vi "v3.vi"() -> ()   [LabVIEW 2015]
uses:
  <vilib>/Utility/miscctls.llb/LVDateTimeRec.ctl
  <vilib>/Analysis/3filter.llb/Filter Passband Type.ctl
  <vilib>/Analysis/8numeric.llb/1D Numeric Integration.vi
  <vilib>/Utility/inputDevices.llb/mouseAcquire.vi
  <vilib>/Utility/inputDevices.llb/closeMouse.vi
  <vilib>/Utility/cursorutil.llb/Set Cursor (Icon Pict).vi
  <vilib>/Analysis/3filter.llb/Butterworth Filter (DBL).vi
  <vilib>/Utility/file.llb/Write Delimited Spreadsheet (DBL).vi
  <vilib>/Analysis/NI_AALBase.lvlib
  <vilib>/Analysis/NI_AALPro.lvlib
panel:
  out "ER":string
  out "TM":string
  out "Vertical (cm/px)":dbl
  out "Horizontal (cm/px)":dbl
  out "Alvo_vertical_px":dbl
  out "Alvo_horizontal_px":dbl
  out "Horizontal_atual_px":i32
  out "Vertical_atual_px":i32
  out "cont6":dbl
  out "cont5":dbl
  out "cont4":dbl
  out "cont2":dbl
  out "cont3":dbl
  out "cont1":dbl
  out "codigo":dbl
  out "Area_acel_1_sub":dbl format="%0.4f"
  out "Area_acel_2_sub":dbl format="%0.4f"
  out "Posicao_final_horizontal":dbl
  out "Posicao_final_Vertical":dbl
  out "Posicao_Hori_2_sub":dbl
  out "Posicao_vert_2_sub":dbl
  out "Deslocamento_Horizontal_fill":dbl[](array[numeric])
  out "Deslocamento_Vertical_fill":dbl[](array[numeric])
  out "Deslocamento_tototal_1_sub":dbl[](array[numeric])
  out "Deslocamento_tototal_2_sub":dbl[](array[numeric])
  out "2_sub_mov(s)":dbl
  out "Fim_da_reposta(s)":dbl format="%#.17g"
  out "Inicio_da_reposta(s)":dbl format="%#.17g"
  out "Apresentacao_do_estimulo(s)":dbl format="%#.17g"
  out "Fim_do_warning(s)":dbl format="%#.17g"
  out "Inicio_do_warning(s)":dbl format="%#.17g"
  out "INICIO(s)":dbl format="%#.17g"
  out "Fim_resp_Cluter":T1
  out "Inicio_da_resposta_Cluter":T1
  out "Apresentacao_do_estimulo_Cluter":T1
  out "Fim_do_warning_Cluter":T1
  out "Inicio_do_warning_Cluter":T1
  out "INICIO_Cluter":T1
  out "x/y":dbl
  out "Fim_do_warning":dbl format="%#.10g"
  out "Inicio_do_warning":dbl format="%#.10g"
  out "Posicao_graus_2_sub":dbl
  out "Posicao_cm_2_sub":dbl
  out "ER_no_2_sub":dbl
  out "Posicao_cm_final":dbl
  out "2_sub_mov":dbl format="%#.10g"
  out "Posicao_graus_final":dbl
  out "Graus":dbl[](array[numeric])
  out "n_correcoes":i32
  out "ref_zero_cross":i32[](array[numeric])
  out "Tempo_relativo_pico":dbl
  out "Tempo_para_o_pico":i32
  out "Pico_velocidade":dbl
  out "Fim_resp":dbl format="%#.10g"
  out "Inicio_da_resposta":dbl format="%#.10g"
  out "Vertical_posicao_px":i32[](array[numeric])
  out "Horizontal_posicao_px":i32[](array[numeric])
  out "Jeark":dbl[](array[numeric])
  out "Deslocamento_Horizontal_bruto":dbl[](array[numeric])
  out "Deslocamento_Vertical_bruto":dbl[](array[numeric])
  out "ref_p_inicial_vertical":dbl
  out "posicao_total":dbl[](array[numeric])
  out "INICIO":dbl format="%#.10g"
  out "Apresentacao_do_estimulo":dbl format="%#.10g"
  out "ref_p_inicial_total":dbl
  out "posicao_horizontal":dbl[](array[numeric])
  out "posicao_vertical":dbl[](array[numeric])
  out "Array_x":dbl[](array[numeric])
  out "ref_t_max":dbl
  out "ref_TR":i32
  out "erro radial (cm)":dbl
  out "meta_precisao":dbl
  out "ref_V_alvo":dbl
  out "ref_H_alvo":dbl
  out "ponto_final":dbl
  out "ref_pont":dbl
  out "Deslocamento_Total__bruto":dbl[](array[numeric])
  out "tentativa":i32
  out "referencia de endereco":path
  out "aceleracao":dbl[](array[numeric])
  out "Velocidade":dbl[](array[numeric])
  out "eixo x":dbl[](array[numeric])
  out "Deslocamento_total_filtrado":dbl[](array[numeric])
  out "cursor":picture
  in  "Tab Control":enum32{"Execucao", "Configuração", "Gráficos"}(tab)
  out "tela":picture
  out "ref_p_inicial_horizontal":dbl
  in  "Cor do ponteiro":u32(colorbox)=14421504
  in  "Cor":u32(colorbox)=197379
  in  "Cor":u32(colorbox)
  in  "Tempo do warning estimulo":u32=1000
  in  "Maior":dbl=3000.0
  in  "menor":dbl=1000.0 format="%#_13g"
  in  "Intervalo entre o fim e o inicio da próxima tentativa":u32=500
  in  "Horizontal (px)":dbl=1366.0
  in  "Horizontal (cm)":dbl=47.2
  in  "Raio":dbl=1.0
  in  "Horizontal":dbl=11.0
  in  "Vertical":dbl=20.0
  in  "Raio":dbl
  in  "Horizontal":dbl
  in  "Vertical":dbl
  in  "Tamanho do ponteiro":dbl=0.2
  in  "Cor":u32(colorbox)
  in  "Raio":dbl
  in  "Horizontal":dbl
  in  "Sincronizar com EEG":bool
  in  "Número de tentativas":i32=10
  in  "Digite aqui o endereço e nome do arquivo":string
  in  "Tempo max  para fechar a tarefa":dbl=1500.0
  in  "Vertical  (cm)":dbl=29.6
  in  "Vertical (px)":dbl=768.0 format="%#_13g"
  in  "Vertical":dbl=20.0 format="%#_13g"
  in  "Horizontal_1":dbl=43.0
  in  "Vertical_1":dbl=20.0
  in  "Raio_1":dbl=0.3
  in  "Horizontal_1":dbl=43.0
  in  "Vertical_1":dbl=20.0 format="%#_13g"
  in  "Cor_1":u32(colorbox)
  in  "Cor_1":u32(colorbox)
  in  "Raio_1":dbl=0.3
  in  "Horizontal_2":dbl
  in  "Vertical_2":dbl
  in  "Raio_2":dbl
  in  "Horizontal_2":dbl
  in  "Vertical_2":dbl=20.0 format="%#_13g"
  in  "Cor_2":u32(colorbox)
  in  "Cor_2":u32(colorbox)
  in  "Raio_2":dbl
  in  "n_tt_1":dbl=10.0
  in  "n_tt_2":dbl
  in  "Horizontal_3":dbl
  in  "Vertical_3":dbl
  in  "Raio_3":dbl
  in  "Horizontal_3":dbl
  in  "Vertical_3":dbl=20.0 format="%#_13g"
  in  "Cor_3":u32(colorbox)
  in  "Cor_3":u32(colorbox)
  in  "Raio_3":dbl
  in  "n_tt_3":dbl
  in  "n_alvos":dbl=1.0
  in  "Horizontal_4":dbl
  in  "Vertical_4":dbl
  in  "Raio_4":dbl
  in  "Horizontal_4":dbl
  in  "Vertical_4":dbl=20.0 format="%#_13g"
  in  "Cor_4":u32(colorbox)
  in  "Cor_4":u32(colorbox)
  in  "Raio_4":dbl
  in  "n_tt_4":dbl
  in  "Raio_5":dbl
  in  "Cor_5":u32(colorbox)
  in  "Cor_5":u32(colorbox)
  in  "Vertical_5":dbl=20.0 format="%#_13g"
  in  "Horizontal_5":dbl
  in  "Raio_5":dbl
  in  "Vertical_5":dbl
  in  "Horizontal_5":dbl
  in  "n_tt_5":dbl
  in  "Raio_6":dbl
  in  "Cor_6":u32(colorbox)
  in  "Cor_6":u32(colorbox)
  in  "Vertical_6":dbl=20.0 format="%#_13g"
  in  "Horizontal_6":dbl
  in  "Raio_6":dbl
  in  "Vertical_6":dbl
  in  "Horizontal_6":dbl
  in  "n_tt_6":dbl
  in  "Tempo max  do tempo de reaçao":dbl=3000.0
  out "Deslocamento":cluster{"X":dbl[], "Y":dbl[]}[](graph) caption="XY Graph"
  out "Velocidade":cluster{"X":dbl[], "Y":dbl[]}[](graph) caption="XY Graph"
  out "Aceleracao":cluster{"X":dbl[], "Y":dbl[]}[](graph) caption="XY Graph"
  out "Jeark":cluster{"X":dbl[], "Y":dbl[]}[](graph) caption="XY Graph"
  out "Tempo de reação":i32
  out "execucao":picture
  out "Tempo de movimento":i32
  out "home":picture
  # "100 h\n500 v"
  # "800 h\n100 v"
  # "Intervalo aleatória entre o prepara e vai"
  # "entre"
  # "Home"
  # "Ponteiro"
  # "Número de alvos"
  # "Posição do alvo 1 - Execução"
  # "Posição do alvo 1 - Preparação"
  # "Horizontal"
  # "Horizontal"
  # "Raio"
  # "Raio"
  # "Número de tentativas do alvo"
  # "Vertical"
  # "Vertical"
  # "Desenvolvido por Tércio Apolinário-Souza"
  # "Posição do alvo 2 - Execução"
  # "Posição do alvo 2 - Preparação"
  # "Horizontal"
  # "Horizontal"
  # "Raio"
  # "Raio"
  # "Número de tentativas do alvo"
  # "Vertical"
  # "Vertical"
  # "Posição do alvo 3 - Preparação"
  # "Posição do alvo 3 - Execução"
  # "Horizontal"
  # "Horizontal"
  # "Raio"
  # "Raio"
  # "Número de tentativas do alvo"
  # "Vertical"
  # "Vertical"
  # "Posição do alvo 4 - Execução"
  # "Posição do alvo 4 - Preparação"
  # "Horizontal"
  # "Horizontal"
  # "Raio"
  # "Raio"
  # "Número de tentativas do alvo"
  # "Vertical"
  # "Vertical"
  # "Posição do alvo 5 - Preparação"
  # "Posição do alvo 5 - Execução"
  # "Horizontal"
  # "Horizontal"
  # "Raio"
  # "Raio"
  # "Número de tentativas do alvo"
  # "Vertical"
  # "Vertical"
  # "Posição do alvo 6 - Preparação"
  # "Posição do alvo 6 - Execução"
  # "Horizontal"
  # "Horizontal"
  # "Raio"
  # "Raio"
  # "Número de tentativas do alvo"
  # "Vertical"
  # "Vertical"
  # "Linger"
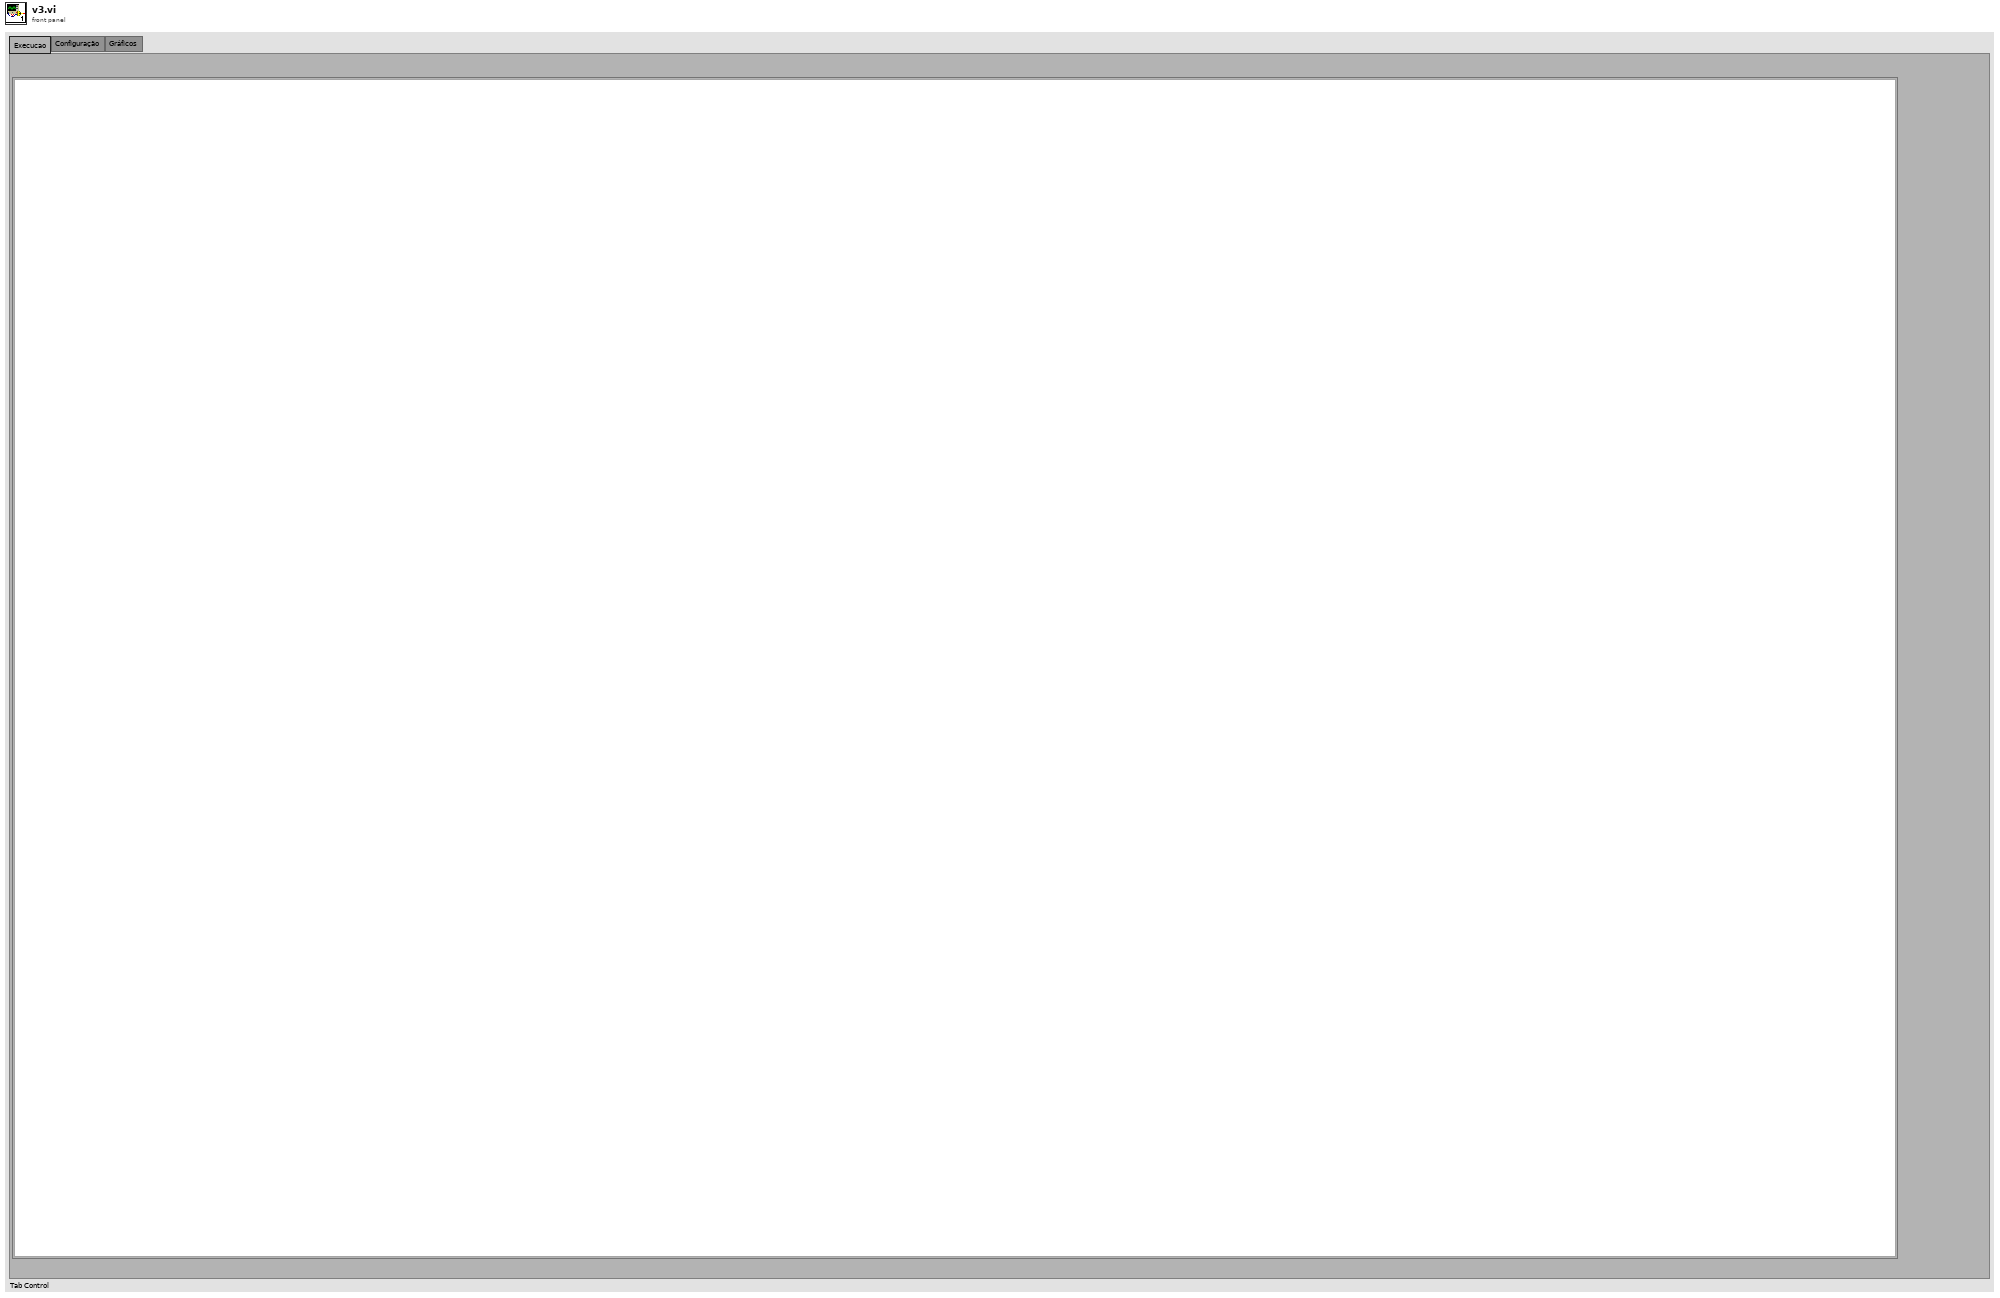
[diagram p1: front panel]
types:
  T1 = typedef "LVDateTimeRec.ctl" = cluster{"fractional second":dbl, "second":i32, "minute":i32, "hour":i32, "day of month":i32, "month":i32, "year":i32, "day of week":i32, "day of year":i32, "DST":i32}
  T2 = typedef "NI_AALBase.lvlib/Filter Passband Type.ctl" = enum32{"Lowpass", "Highpass", "Bandpass", "Bandstop"}
  T3 = cluster{"button 1":bool, "button 2":bool, "button 3":bool, "button 4":bool}
  T4 = cluster{"Horizontal":i32, "Vertical":i32, "Scrolling":i32}
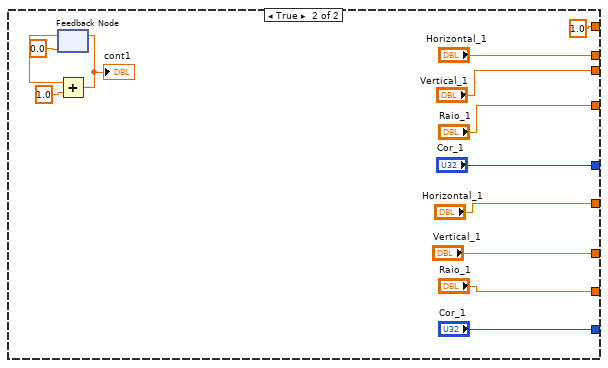
[diagram p4: hidden frame]
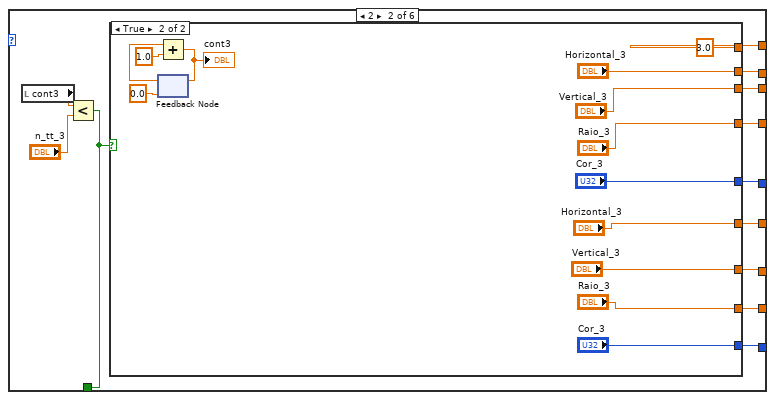
[diagram p5: hidden frame]
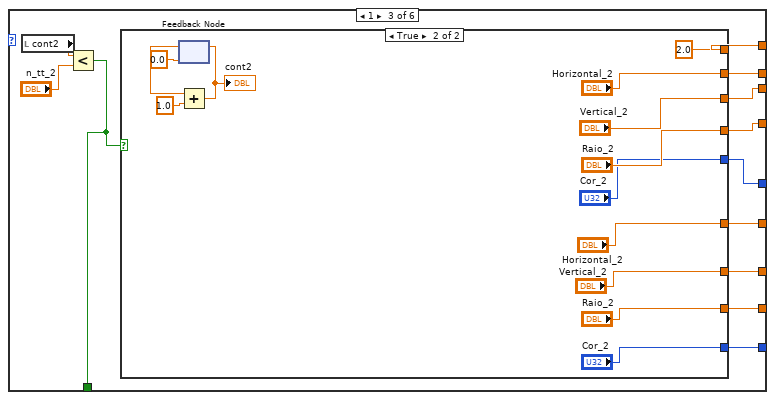
[diagram p7: hidden frame]
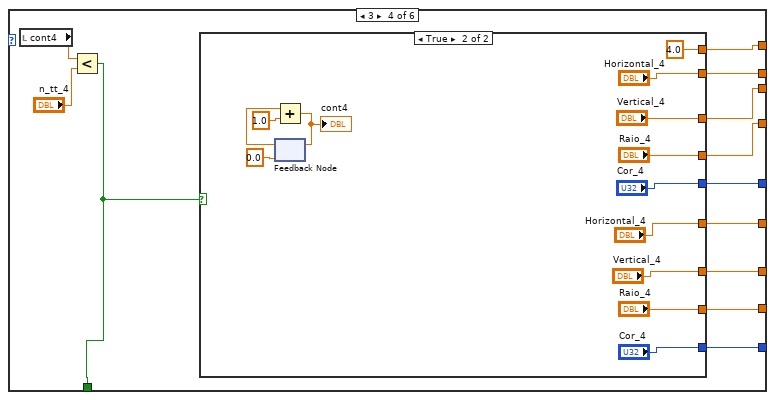
[diagram p9: hidden frame]
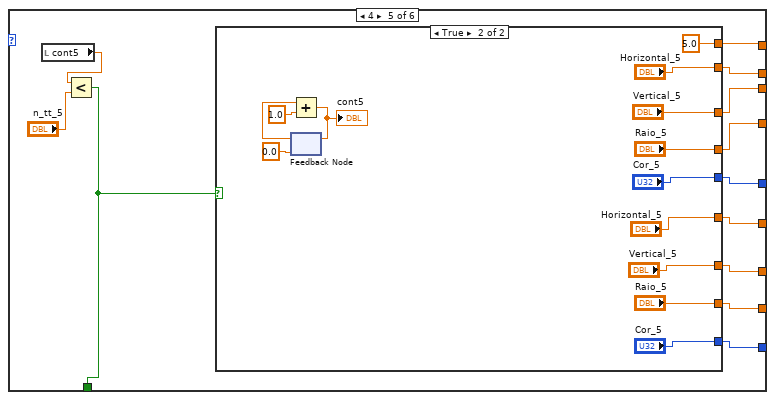
[diagram p11: hidden frame]
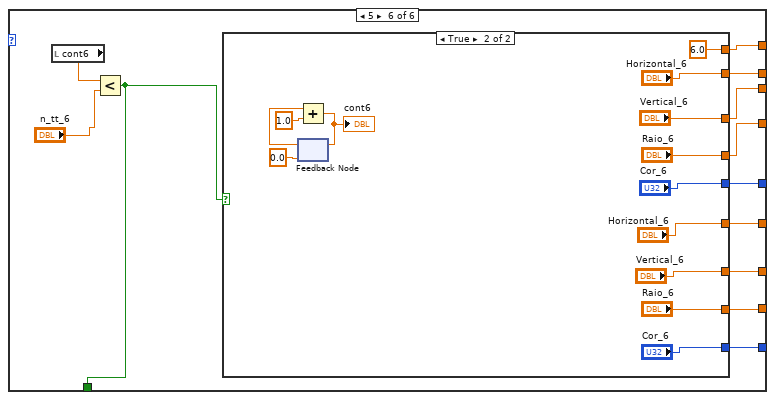
[diagram p13: hidden frame]
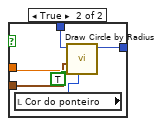
[diagram p20: hidden frame]
diagram:
  w10 = 0.0 ("cont1")
  # "esquerda\ncima\ndireita\nbaixo"
  n1 = local write "cont4"(w10) -> ()
  n2 = local write "cont3"(w10) -> ()
  n3 = local write "cont5"(w10) -> ()
  n4 = local write "cont6"(w10) -> ()
  n5 = local write "cont1"(w10) -> ()
  n6 = local write "cont2"(w10) -> ()
  n7 = for {
    N: "Número de tentativas" -> [_]
    tunnel: [w126] -> w81 mode=indexing
    tunnel: [w125] -> w79 mode=indexing
    tunnel: [w124] -> w77 mode=indexing
    tunnel: [w123] -> w75 mode=indexing
    tunnel: [w122] -> w73 mode=indexing
    tunnel: [w121] -> w71 mode=indexing
    tunnel: [w120] -> w69 mode=indexing
    tunnel: [w119] -> w67 mode=indexing
    tunnel: [w118] -> w65 mode=indexing
    tunnel: [w117] -> w63 mode=indexing
    tunnel: [w116] -> w61 mode=indexing
    tunnel: [w115] -> w59 mode=indexing
    tunnel: [w114] -> w57 mode=indexing
    tunnel: [w113] -> w55 mode=indexing
    tunnel: [w112] -> w52 mode=indexing
    tunnel: [w111] -> w51 mode=indexing
    tunnel: [w110] -> w48 mode=indexing
    tunnel: [w109] -> w47 mode=indexing
    tunnel: [w108] -> w45 mode=indexing
    tunnel: [w107] -> w43 mode=indexing
    tunnel: [w106] -> w41 mode=indexing
    tunnel: [w105] -> w39 mode=indexing
    tunnel: [w104] -> w37 mode=indexing
    tunnel: [w103] -> w35 mode=indexing
    tunnel: [w102] -> w32 mode=indexing
    tunnel: [w101] -> w30 mode=indexing
    tunnel: [w100] -> w29 mode=indexing
    tunnel: [w99] -> w27 mode=indexing
    tunnel: [w98] -> w26 mode=indexing
    tunnel: [w97] -> w24 mode=indexing
    tunnel: [w96] -> w22 mode=indexing
    tunnel: [w95] -> w13 mode=indexing
    tunnel: [w94] -> w19 mode=indexing
    tunnel: [w93] -> w17 mode=indexing
    tunnel: [w92] -> w16 mode=indexing
    tunnel: [w91] -> w9 mode=indexing
    tunnel: [w90] -> w8 mode=indexing
    tunnel: [w89] -> w6 mode=indexing
    tunnel: [w88] -> w4 mode=indexing
    tunnel: [w87] -> w2 mode=indexing
    i -> [w141]
    n8 = Increment(x=w141) -> (x+1=→"tentativa":i32)
    n9 = flat-sequence {
      tunnel: w141 -> [w144]
      tunnel: [w508] -> w139
      tunnel: [w507] -> w134
      tunnel: w139 -> [w614]
      tunnel: [w609] -> w136
      tunnel: [w608] -> w135
      tunnel: w134 -> [w617]
      tunnel: [w607] -> w133
      tunnel: [w680] -> w138
      tunnel: w136 -> [w669]
      tunnel: w135 -> [w663]
      tunnel: w133 -> [w662]
      tunnel: [w660] -> w132
      tunnel: [w661] -> w130
      tunnel: w138 -> [w699]
      tunnel: [w699] -> w137
      tunnel: w132 -> [w686]
      tunnel: [w686] -> w131
      tunnel: w130 -> [w684]
      tunnel: [w684] -> w129
      tunnel: w137 -> [w731]
      tunnel: w131 -> [w728]
      tunnel: w129 -> [w725]
      tunnel: [w864] -> w128
      tunnel: [w864] -> w127
      tunnel: w128 -> [w900]
      tunnel: w127 -> [w912]
      tunnel: [w1109] -> w126
      tunnel: [w1108] -> w125
      tunnel: [w1107] -> w124
      tunnel: [w1106] -> w123
      tunnel: [w1105] -> w122
      tunnel: [w1104] -> w121
      tunnel: [w1103] -> w120
      tunnel: [w1102] -> w119
      tunnel: [w1101] -> w118
      tunnel: [w1100] -> w117
      tunnel: [w1099] -> w116
      tunnel: [w1098] -> w115
      tunnel: [w1097] -> w114
      tunnel: [w1096] -> w113
      tunnel: [w1095] -> w112
      tunnel: [w1094] -> w111
      tunnel: [w1093] -> w110
      tunnel: [w1092] -> w109
      tunnel: [w1091] -> w108
      tunnel: [w1090] -> w107
      tunnel: [w1089] -> w106
      tunnel: [w1088] -> w105
      tunnel: [w1087] -> w104
      tunnel: [w1086] -> w103
      tunnel: [w1085] -> w102
      tunnel: [w1084] -> w101
      tunnel: [w1083] -> w100
      tunnel: [w1082] -> w99
      tunnel: [w1081] -> w98
      tunnel: [w1080] -> w97
      tunnel: [w1079] -> w96
      tunnel: [w1069] -> w95
      tunnel: [w1066] -> w94
      tunnel: [w1078] -> w93
      tunnel: [w1077] -> w92
      tunnel: [w1065] -> w91
      tunnel: [w1064] -> w90
      tunnel: [w1063] -> w89
      tunnel: [w1062] -> w88
      tunnel: [w1061] -> w87
      frame #0 {
        n10 = Equal?(x=w144, y=0) -> (x = y?=w148:bool)
        n11 = And(x="Sincronizar com EEG", y=w148) -> (x .and. y?=w146:bool)
        n12 = case shown="True" w146 {
          frame False {
          }
          frame True {
            n13 = call <vilib>:"Initialize Mouse.vi"() -> ("error out"=w150:errorcluster, "device ID"=w151:refnum<k1>)  [unwired: 10 in]
            n14 = while {
              tunnel: w151 -> [w157]
              tunnel: w150 -> [w156]
              tunnel: enum16{"RELATIVE", "ABSOLUTE"}."ABSOLUTE" ("key mode") -> [w155]
              stop <- w153 stop-if-true
              n15 = call-poly <vilib>:"Acquire Input Data.vi"("device ID"=w157, "key mode"=w155, "error in (no error)"=w156) -> ("button info"=w154:T3)  [unwired: 13 in, 3 out]
              n16 = Unbundle(w154) -> ("button 1"=w152:bool)  [unwired: 3 out]
              n17 = case shown="True" w152 {
                tunnel: [_ TRUE] -> w153
                frame False {
                }
                frame True {
                  n18 = Get Date/Time In Seconds() -> (seconds since 1Jan1904=w159:timestamp)
                  n19 = Format Date/Time String(time format string (%c)="%H%M%S%4u", seconds (now)=w159) -> (date/time string=w161:string)  [unwired: 1 in]
                  n20 = Fract/Exp String To Number(use system decimal point (T)=TRUE, string=w161) -> (number=→"INICIO":dbl)  [unwired: 2 in, 1 out]
                  n21 = Seconds To Date/Time(time stamp (now)=w159) -> (date time rec=→"INICIO_Cluter":T1)  [unwired: 1 in]
                }
              }
            }
          }
        }
        n22 = property on="TM" class="Str"("Visible"=FALSE) -> ()  [unwired: 2 in, 2 out]
        n23 = property on="ER" class="Str"("Visible"=FALSE) -> ()  [unwired: 2 in, 2 out]
      }
      frame #1 {
        n24 = Divide(x="Vertical  (cm)", y="Vertical (px)") -> (x/y=→"Vertical (cm/px)":dbl)
        n25 = Divide(x="Horizontal (cm)", y="Horizontal (px)") -> (x/y=→"Horizontal (cm/px)":dbl)
      }
      frame #2 {
        # "execucao"
        # "Preparacao"
        # "Selecioar alvo"
        n26 = while {
          tunnel: [w189] -> w179
          tunnel: [w188] -> w178
          tunnel: [w187] -> w177
          tunnel: [w186] -> w176
          tunnel: [w185] -> w172
          tunnel: [w184] -> w171
          tunnel: [w183] -> w175
          tunnel: [w182] -> w174
          tunnel: [w180] -> w173
          stop <- w195 stop-if-true
          n27 = Random Number (0-1)() -> (number: 0 to 1=w193:dbl)
          n28 = Multiply(x=w193, y=100.0) -> (x*y=w192:dbl)
          n29 = To Byte Integer(number=w192) -> (8bit integer=w191:i8)
          n30 = Quotient & Remainder(x=w191, y="n_alvos") -> (x-y*floor(x/y)=w190:dbl)  [unwired: 1 out]
          n31 = case shown="0, Default" w190 {
            tunnel: [w207 w232 w257 w279 w307 w328] -> w180
            tunnel: [w205 w230 w255 w281 w297 w330] -> w195
            tunnel: [w204 w229 w254 w278 w306 w329] -> w189
            tunnel: [w203 w228 w253 w277 w305 w327] -> w188
            tunnel: [w202 w227 w252 w276 w304 w326] -> w187
            tunnel: [w201 w226 w251 w275 w303 w325] -> w186
            tunnel: [w200 w225 w250 w274 w302 w324] -> w185
            tunnel: [w199 w224 w249 w273 w301 w323] -> w184
            tunnel: [w198 w223 w248 w272 w300 w322] -> w183
            tunnel: [w197 w222 w247 w271 w299 w321] -> w182
            frame 0, Default {
              n32 = local read "cont1"() -> (w206:dbl)
              n33 = Less?(x=w206, y="n_tt_1") -> (x < y?=w205:bool)
              n34 = case shown="False" w205 {
                tunnel: [_ 1.0] -> w207
                tunnel: [_ "Horizontal_1"] -> w204
                tunnel: [_ "Vertical_1"] -> w203
                tunnel: [_ "Raio_1"] -> w202
                tunnel: [_ "Cor_1"] -> w201
                tunnel: [_ "Horizontal_1"] -> w200
                tunnel: [_ "Vertical_1"] -> w199
                tunnel: [_ "Raio_1"] -> w198
                tunnel: [_ "Cor_1"] -> w197
                frame False {
                }
                frame True {
                  n35 = feedback #1(0.0) -> (w219:dbl)
                  n36 = Add(x=w219, y=1.0) -> (x+y=w216:dbl)
                  "cont1" <- w216
                  n37 = feedback-in #1(w216) -> ()
                }
              }
            }
            frame 2 {
              n38 = local read "cont3"() -> (w231:dbl)
              n39 = Less?(x=w231, y="n_tt_3") -> (x < y?=w230:bool)
              n40 = case shown="True" w230 {
                tunnel: [_ 3.0] -> w232
                tunnel: [_ "Horizontal_3"] -> w229
                tunnel: [_ "Vertical_3"] -> w228
                tunnel: [_ "Raio_3"] -> w227
                tunnel: [_ "Cor_3"] -> w226
                tunnel: [_ "Horizontal_3"] -> w225
                tunnel: [_ "Vertical_3"] -> w224
                tunnel: [_ "Raio_3"] -> w223
                tunnel: [_ "Cor_3"] -> w222
                frame False {
                }
                frame True {
                  n41 = feedback #2(0.0) -> (w243:dbl)
                  n42 = Add(x=w243, y=1.0) -> (x+y=w244:dbl)
                  "cont3" <- w244
                  n43 = feedback-in #2(w244) -> ()
                }
              }
            }
            frame 1 {
              n44 = local read "cont2"() -> (w256:dbl)
              n45 = Less?(x=w256, y="n_tt_2") -> (x < y?=w255:bool)
              n46 = case shown="True" w255 {
                tunnel: [_ 2.0] -> w257
                tunnel: [_ "Horizontal_2"] -> w254
                tunnel: [_ "Vertical_2"] -> w253
                tunnel: [_ "Raio_2"] -> w252
                tunnel: [_ "Cor_2"] -> w251
                tunnel: [_ "Horizontal_2"] -> w250
                tunnel: [_ "Vertical_2"] -> w249
                tunnel: [_ "Raio_2"] -> w248
                tunnel: [_ "Cor_2"] -> w247
                frame False {
                }
                frame True {
                  n47 = feedback #3(0.0) -> (w268:dbl)
                  n48 = Add(x=w268, y=1.0) -> (x+y=w269:dbl)
                  "cont2" <- w269
                  n49 = feedback-in #3(w269) -> ()
                }
              }
            }
            frame 3 {
              n50 = local read "cont4"() -> (w280:dbl)
              n51 = Less?(x=w280, y="n_tt_4") -> (x < y?=w281:bool)
              n52 = case shown="True" w281 {
                tunnel: [_ 4.0] -> w279
                tunnel: [_ "Horizontal_4"] -> w278
                tunnel: [_ "Vertical_4"] -> w277
                tunnel: [_ "Raio_4"] -> w276
                tunnel: [_ "Cor_4"] -> w275
                tunnel: [_ "Horizontal_4"] -> w274
                tunnel: [_ "Vertical_4"] -> w273
                tunnel: [_ "Raio_4"] -> w272
                tunnel: [_ "Cor_4"] -> w271
                frame False {
                }
                frame True {
                  n53 = feedback #4(0.0) -> (w294:dbl)
                  n54 = Add(x=w294, y=1.0) -> (x+y=w295:dbl)
                  "cont4" <- w295
                  n55 = feedback-in #4(w295) -> ()
                }
              }
            }
            frame 4 {
              n56 = local read "cont5"() -> (w296:dbl)
              n57 = Less?(x=w296, y="n_tt_5") -> (x < y?=w297:bool)
              n58 = case shown="True" w297 {
                tunnel: [_ 5.0] -> w307
                tunnel: [_ "Horizontal_5"] -> w306
                tunnel: [_ "Vertical_5"] -> w305
                tunnel: [_ "Raio_5"] -> w304
                tunnel: [_ "Cor_5"] -> w303
                tunnel: [_ "Horizontal_5"] -> w302
                tunnel: [_ "Vertical_5"] -> w301
                tunnel: [_ "Raio_5"] -> w300
                tunnel: [_ "Cor_5"] -> w299
                frame False {
                }
                frame True {
                  n59 = feedback #5(0.0) -> (w319:dbl)
                  n60 = Add(x=w319, y=1.0) -> (x+y=w320:dbl)
                  "cont5" <- w320
                  n61 = feedback-in #5(w320) -> ()
                }
              }
            }
            frame 5 {
              n62 = local read "cont6"() -> (w331:dbl)
              n63 = Less?(x=w331, y="n_tt_6") -> (x < y?=w330:bool)
              n64 = case shown="True" w330 {
                tunnel: [_ 6.0] -> w328
                tunnel: [_ "Horizontal_6"] -> w329
                tunnel: [_ "Vertical_6"] -> w327
                tunnel: [_ "Raio_6"] -> w326
                tunnel: [_ "Cor_6"] -> w325
                tunnel: [_ "Horizontal_6"] -> w324
                tunnel: [_ "Vertical_6"] -> w323
                tunnel: [_ "Raio_6"] -> w322
                tunnel: [_ "Cor_6"] -> w321
                frame False {
                }
                frame True {
                  n65 = feedback #6(0.0) -> (w344:dbl)
                  n66 = Add(x=w344, y=1.0) -> (x+y=w345:dbl)
                  "cont6" <- w345
                  n67 = feedback-in #6(w345) -> ()
                }
              }
            }
          }
        }
        "codigo" <- w173
        n68 = local write "Horizontal"(w179) -> ()
        n69 = local write "Vertical"(w178) -> ()
        n70 = local write "Horizontal"(w172) -> ()
        n71 = local write "Raio"(w175) -> ()
        n72 = local write "Cor"(w176) -> ()
        n73 = local write "Vertical"(w171) -> ()
        n74 = local write "Raio"(w177) -> ()
        n75 = local write "Cor"(w174) -> ()
      }
      frame #3 {
        # "Preparação"
        n76 = call <vilib>:"Initialize Mouse.vi"() -> ("error out"=w348:errorcluster, "device ID"=w349:refnum<k1>)  [unwired: 10 in]
        n77 = while {
          tunnel: w349 -> [w401]
          tunnel: w348 -> [w394]
          tunnel: [w376] -> w347
          tunnel: [w395] -> w346
          stop <- w396 stop-if-true
          # "Alvo 1"
          n78 = local read "Vertical  (cm)"() -> (w374:dbl)
          n79 = local read "Horizontal (cm/px)"() -> (w353:dbl)
          n80 = call-poly <vilib>:"Acquire Input Data.vi"("device ID"=w401, "error in (no error)"=w394) -> ("device ID"=w376:refnum<k1>, "axis info"=w400:T4, "error out"=w395:errorcluster)  [unwired: 14 in, 1 out]
          n81 = Subtract(x=w374, y="Vertical") -> (x-y=w373:dbl)
          n82 = Divide(x=w373, y=w353) -> (x/y=w352:dbl)
          n83 = Unbundle By Name(w400) -> ("Vertical"=w368:i32, "Horizontal"=w371:i32)
          n84 = Divide(x="Horizontal", y=w353) -> (x/y=w377:dbl)
          n85 = Divide(x="Raio", y=w353) -> (x/y=w360:dbl)
          "x/y" <- w360
          n86 = Bundle(w377, w352) -> (w384:cluster{dbl, dbl})  [unwired: 1 in]
          n87 = Quotient & Remainder(x=w377, y=1.0) -> (floor(x/y)=w370:dbl)  [unwired: 1 out]
          n88 = Quotient & Remainder(x=w352, y=1.0) -> (floor(x/y)=w367:dbl)  [unwired: 1 out]
          n89 = call <vilib>:"Draw Circle by Radius.vi"("color(black)"="Cor", "fill?(F)"=TRUE, "pixel center"=w384, "radius"=w360) -> ("new picture"=w385:picture)  [unwired: 7 in]
          "home" <- w385
          n90 = Subtract(x=w371, y=w370) -> (x-y=w369:dbl)
          n91 = local read "Horizontal (cm/px)"() -> (w386:dbl)
          n92 = Subtract(x=w368, y=w367) -> (x-y=w366:dbl)
          n93 = Absolute Value(x=w369) -> (abs(x)=w363:dbl)
          n94 = local read "Vertical  (cm)"() -> (w375:dbl)
          n95 = local read "Vertical"() -> (w356:dbl)
          n96 = local read "Horizontal (cm/px)"() -> (w381:dbl)
          n97 = local read "Raio"() -> (w357:dbl)
          n98 = local read "Horizontal"() -> (w358:dbl)
          n99 = Absolute Value(x=w366) -> (abs(x)=w362:dbl)
          n100 = Divide(x=w360, y=2.0) -> (x/y=w359:dbl)
          n101 = Less Or Equal?(x=w362, y=w359) -> (x <= y?=w364:bool)
          n102 = Less Or Equal?(x=w363, y=w359) -> (x <= y?=w365:bool)
          n103 = Bundle("Horizontal"=w371, "Vertical"=w368) -> (w399:cluster{"Horizontal":i32, "Vertical":i32})  [unwired: 1 in]
          n104 = Subtract(x=w375, y=w356) -> (x-y=w372:dbl)
          n105 = And(x=w364, y=w365) -> (x .and. y?=w396:bool)
          n106 = Divide(x=w372, y=w386) -> (x/y=w350:dbl)
          "ref_V_alvo" <- w350
          n107 = Divide(x=w357, y=w386) -> (x/y=w390:dbl)
          n108 = Divide(x=w358, y=w386) -> (x/y=w351:dbl)
          "ref_H_alvo" <- w351
          n109 = Divide(x="Tamanho do ponteiro", y=w381) -> (x/y=w380:dbl)
          "ref_pont" <- w380
          n110 = Bundle(w351, w350) -> (w387:cluster{dbl, dbl})  [unwired: 1 in]
          n111 = local read "Cor"() -> (w355:u32)
          n112 = call <vilib>:"Draw Circle by Radius.vi"("color(black)"=w355, "fill?(F)"=TRUE, "pixel center"=w387, "radius"=w390, "picture"=w385) -> ("new picture"=w389:picture)  [unwired: 6 in]
          "cursor" <- w389
          n113 = call <vilib>:"Draw Circle by Radius.vi"("color(black)"="Cor do ponteiro", "fill?(F)"=TRUE, "pixel center"=w399, "radius"=w380, "picture"=w389) -> ("new picture"=→"tela":picture)  [unwired: 6 in]
        }
        n114 = call-poly <vilib>:"Close Input Device.vi"("error in (no error)"=w346, "device ID"=w347) -> ()  [unwired: 8 in, 1 out]
      }
      frame #4 {
      }
      frame #5 {
        n115 = case shown="True" TRUE {
          frame False {
          }
          frame True {
            n116 = Get Date/Time In Seconds() -> (seconds since 1Jan1904=w409:timestamp)
            n117 = Format Date/Time String(time format string (%c)="%H%M%S%4u", seconds (now)=w409) -> (date/time string=w411:string)  [unwired: 1 in]
            n118 = Fract/Exp String To Number(use system decimal point (T)=TRUE, string=w411) -> (number=→"Inicio_do_warning":dbl)  [unwired: 2 in, 1 out]
            n119 = Seconds To Date/Time(time stamp (now)=w409) -> (date time rec=→"Inicio_do_warning_Cluter":T1)  [unwired: 1 in]
          }
        }
        n120 = Wait (ms)(milliseconds to wait="Tempo do warning estimulo") -> ()  [unwired: 1 out]
        n121 = call <vilib>:"Beep.vi"("use system alert? (T)"=FALSE, "duration (msec)"=u32 200, "frequency (Hz)"=u32 500) -> ()  [unwired: 9 in]
      }
      frame #6 {
        # "intervalo entre 1 a 3 segundo"
        # "Isso serve para apagar"
        n122 = case shown="True" TRUE {
          frame False {
          }
          frame True {
            n123 = Get Date/Time In Seconds() -> (seconds since 1Jan1904=w423:timestamp)
            n124 = Format Date/Time String(time format string (%c)="%H%M%S%4u", seconds (now)=w423) -> (date/time string=w426:string)  [unwired: 1 in]
            n125 = Fract/Exp String To Number(use system decimal point (T)=TRUE, string=w426) -> (number=→"Fim_do_warning":dbl)  [unwired: 2 in, 1 out]
            n126 = Seconds To Date/Time(time stamp (now)=w423) -> (date time rec=→"Fim_do_warning_Cluter":T1)  [unwired: 1 in]
          }
        }
        n127 = Random Number (0-1)() -> (number: 0 to 1=w416:dbl)
        n128 = Subtract(x="Maior", y=1.0) -> (x-y=w421:dbl)
        n129 = call <vilib>:"Draw Circle by Radius.vi"() -> ("new picture"=w415:picture)  [unwired: 11 in]
        n130 = Multiply(x=w421, y=w416) -> (x*y=w417:dbl)
        n131 = Add(x=w417, y="menor") -> (x+y=w422:dbl)
        n132 = local write "tela"(w415) -> ()
        n133 = Wait (ms)(milliseconds to wait=w422) -> ()  [unwired: 1 out]
      }
      frame #7 {
        w437 = dbl[] [0.0]
        # "Tempo reação"
        n134 = call <vilib>:"Initialize Mouse.vi"() -> ("error out"=w439:errorcluster, "device ID"=w440:refnum<k1>)  [unwired: 10 in]
        n135 = case shown="True" TRUE {
          frame False {
          }
          frame True {
            n136 = Get Date/Time In Seconds() -> (seconds since 1Jan1904=w441:timestamp)
            n137 = Format Date/Time String(time format string (%c)="%H%M%S%4u", seconds (now)=w441) -> (date/time string=w444:string)  [unwired: 1 in]
            n138 = Fract/Exp String To Number(use system decimal point (T)=TRUE, string=w444) -> (number=→"Apresentacao_do_estimulo":dbl)  [unwired: 2 in, 1 out]
            n139 = Seconds To Date/Time(time stamp (now)=w441) -> (date time rec=→"Apresentacao_do_estimulo_Cluter":T1)  [unwired: 1 in]
          }
        }
        n140 = while {
          tunnel: w440 -> [w496]
          tunnel: w439 -> [w495]
          tunnel: [w492] -> w433
          tunnel: [w494] -> w438
          shift-right: [w491] -> _
          shift-left: w437 -> [w490]
          shift-left: w437 -> [w487]
          tunnel: [w452] -> w435
          i -> [w452]
          stop <- w453 stop-if-true
          n141 = local read "Horizontal (cm/px)"() -> (w475:dbl)
          n142 = local read "Horizontal"() -> (w459:dbl)
          n143 = local read "Vertical  (cm)"() -> (w461:dbl)
          n144 = local read "Vertical"() -> (w458:dbl)
          n145 = Divide(x="Tempo max  do tempo de reaçao", y=10.0) -> (x/y=w449:dbl)
          n146 = call-poly <vilib>:"Acquire Input Data.vi"("device ID"=w496, "error in (no error)"=w495) -> ("device ID"=w492:refnum<k1>, "axis info"=w465:T4, "error out"=w494:errorcluster)  [unwired: 14 in, 1 out]
          n147 = Subtract(x=w452, y=2) -> (x-y=w488:i32)
          n148 = Subtract(x=w461, y=w458) -> (x-y=w460:dbl)
          n149 = local read "Raio"() -> (w456:dbl)
          n150 = Divide(x=w460, y=w475) -> (x/y=w447:dbl)
          "Alvo_vertical_px" <- w447
          n151 = Divide(x=w459, y=w475) -> (x/y=w448:dbl)
          "Alvo_horizontal_px" <- w448
          n152 = Unbundle By Name(w465) -> ("Vertical"=w468:i32, "Horizontal"=w469:i32)
          n153 = Wait Until Next ms Multiple(millisecond multiple=u32 10) -> ()  [unwired: 1 out]
          n154 = Index Array(array=w487, index=w488) -> (element=w484:dbl)
          n155 = Index Array(array=w490, index=w452) -> (element=w485:dbl)
          n156 = local read "home"() -> (w474:picture)
          n157 = Bundle(w448, w447) -> (w477:cluster{dbl, dbl})  [unwired: 1 in]
          n158 = Divide(x=w456, y=w475) -> (x/y=w476:dbl)
          n159 = Subtract(x=w485, y=w484) -> (x-y=w483:dbl)
          n160 = local read "Cor"() -> (w457:u32)
          n161 = feedback #7(0.0) -> (w482:dbl)
          n162 = Not Equal To 0?(x=w483) -> (x != 0?=w479:bool)
          n163 = Square(x=w468) -> (x^2=w493:i32)
          n164 = Square(x=w469) -> (x^2=w464:i32)
          n165 = case shown="True" w479 {
            tunnel: [_ w498] -> w481
            tunnel: w482 -> [_ w500]
            tunnel: [_ w499] -> w454
            frame False {
            }
            frame True {
              n166 = Increment(x=w500) -> (x+1=w498:dbl)
              n167 = Greater Or Equal?(x=w498, y=3.0) -> (x >= y?=w499:bool)
            }
          }
          n168 = feedback-in #7(w481) -> ()
          n169 = call <vilib>:"Draw Circle by Radius.vi"("color(black)"=w457, "fill?(F)"=TRUE, "pixel center"=w477, "radius"=w476, "picture"=w474) -> ("new picture"=w473:picture)  [unwired: 6 in]
          "execucao" <- w473
          n170 = Add(x=w493, y=w464) -> (x+y=w463:i32)
          n171 = local read "ref_pont"() -> (w471:dbl)
          n172 = Square Root(x=w463) -> (sqrt(x)=w462:dbl)
          n173 = Bundle("Horizontal"=w469, "Vertical"=w468) -> (w470:cluster{"Horizontal":i32, "Vertical":i32})  [unwired: 1 in]
          n174 = Greater?(x=w452, y=w449) -> (0:w455:bool)
          n175 = Or(x=w454, y=w455) -> (x .or. y?=w453:bool)
          n176 = Insert Into Array(array=w490, new element=w462) -> (w491:dbl[])  [unwired: 1 in]
          n177 = local read "Cor do ponteiro"() -> (w466:u32)
          n178 = call <vilib>:"Draw Circle by Radius.vi"("color(black)"=w466, "fill?(F)"=TRUE, "pixel center"=w470, "radius"=w471, "picture"=w473) -> ("new picture"=w472:picture)  [unwired: 6 in]
          n179 = local write "tela"(w472) -> ()
          "ref_TR" <- w452
        }
        n180 = call <vilib>:"Beep.vi"("use system alert? (T)"=FALSE, "duration (msec)"=u32 200, "frequency (Hz)"=u32 700) -> ()  [unwired: 9 in]
        n181 = Multiply(x=w435, y=10) -> (x*y=→"Tempo de reação":i32)
        n182 = call-poly <vilib>:"Close Input Device.vi"("error in (no error)"=w438, "device ID"=w433) -> ()  [unwired: 8 in, 1 out]
      }
      frame #8 {
        n183 = local read "ref_TR"() -> (w504:i32)
        n184 = Divide(x="Tempo max  para fechar a tarefa", y=10.0) -> (x/y=w503:dbl)
        n185 = Subtract(x=w503, y=w504) -> (x-y=w505:dbl)
        n186 = Absolute Value(x=w505) -> (abs(x)=→"ref_t_max":dbl)
      }
      frame #9 {
        w510 = i32[] [0]
        w519 = dbl[] [0.0]
        # "Execução"
        n187 = case shown="True" TRUE {
          frame False {
          }
          frame True {
            n188 = Get Date/Time In Seconds() -> (seconds since 1Jan1904=w522:timestamp)
            n189 = Format Date/Time String(time format string (%c)="%H%M%S%4u", seconds (now)=w522) -> (date/time string=w525:string)  [unwired: 1 in]
            n190 = Fract/Exp String To Number(use system decimal point (T)=TRUE, string=w525) -> (number=→"Inicio_da_resposta":dbl)  [unwired: 2 in, 1 out]
            n191 = Seconds To Date/Time(time stamp (now)=w522) -> (date time rec=→"Inicio_da_resposta_Cluter":T1)  [unwired: 1 in]
          }
        }
        n192 = call <vilib>:"Initialize Mouse.vi"() -> ("error out"=w515:errorcluster, "device ID"=w516:refnum<k1>)  [unwired: 10 in]
        n193 = while {
          tunnel: w516 -> [w569]
          tunnel: w515 -> [w573]
          tunnel: [w572] -> w521
          tunnel: [w570] -> w520
          shift-right: [w547] -> _
          shift-left: w519 -> [w554]
          shift-left: w519 -> [w564]
          tunnel: [w542] -> w514
          shift-right: [w549] -> w511
          shift-left: w519 -> [w548]
          shift-right: [w540] -> w507
          shift-left: w510 -> [w539]
          shift-right: [w536] -> w508
          shift-left: w510 -> [w535]
          i -> [w542]
          stop <- w543 stop-if-true
          n194 = call-poly <vilib>:"Acquire Input Data.vi"("device ID"=w569, "error in (no error)"=w573) -> ("device ID"=w570:refnum<k1>, "axis info"=w571:T4, "error out"=w572:errorcluster)  [unwired: 14 in, 1 out]
          n195 = Subtract(x=w542, y=2) -> (x-y=w566:i32)
          n196 = Wait Until Next ms Multiple(millisecond multiple=u32 10) -> ()  [unwired: 1 out]
          n197 = Index Array(array=w564, index=w566) -> (element=w563:dbl)
          n198 = Index Array(array=w554, index=w542) -> (element=w552:dbl)
          n199 = Unbundle By Name(w571) -> ("Vertical"=w538:i32, "Horizontal"=w534:i32)
          "Vertical_atual_px" <- w538
          "Horizontal_atual_px" <- w534
          n200 = local read "ref_pont"() -> (w529:dbl)
          n201 = Subtract(x=w552, y=w563) -> (x-y=w553:dbl)
          n202 = feedback #8(0.0) -> (w561:dbl)
          n203 = Equal To 0?(x=w553) -> (x = 0?=w559:bool)
          n204 = local read "execucao"() -> (w530:picture)
          n205 = Square(x=w538) -> (x^2=w568:i32)
          n206 = Square(x=w534) -> (x^2=w567:i32)
          n207 = case shown="True" w559 {
            tunnel: [_ w583] -> w562
            tunnel: w561 -> [_ w584]
            tunnel: [_ w582] -> w558
            frame False {
            }
            frame True {
              n208 = Increment(x=w584) -> (x+1=w583:dbl)
              n209 = Greater Or Equal?(x=w583, y=8.0) -> (x >= y?=w582:bool)
            }
          }
          n210 = feedback-in #8(w562) -> ()
          n211 = Greater?(x=w542, y=3) -> (0:w557:bool)
          n212 = Add(x=w568, y=w567) -> (x+y=w541:i32)
          n213 = local read "ref_t_max"() -> (w545:dbl)
          n214 = Bundle("Horizontal"=w534, "Vertical"=w538) -> (w531:cluster{"Horizontal":i32, "Vertical":i32})  [unwired: 1 in]
          n215 = Square Root(x=w541) -> (sqrt(x)=w537:dbl)
          n216 = Multiply(x=w542, y=0.01) -> (x*y=w551:dbl)
          n217 = case shown="False" FALSE {
            tunnel: [w574 w578] -> w532
            tunnel: w531 -> [_ w577]
            tunnel: w530 -> [_ w576]
            tunnel: w529 -> [_ w575]
            frame False {
              n218 = call <vilib>:"Draw Circle by Radius.vi"() -> ("new picture"=w574:picture)  [unwired: 11 in]
            }
            frame True {
              n219 = local read "Cor do ponteiro"() -> (w580:u32)
              n220 = call <vilib>:"Draw Circle by Radius.vi"("color(black)"=w580, "fill?(F)"=TRUE, "pixel center"=w577, "radius"=w575, "picture"=w576) -> ("new picture"=w578:picture)  [unwired: 6 in]
            }
          }
          n221 = Insert Into Array(array=w554, new element=w537) -> (w547:dbl[])  [unwired: 1 in]
          n222 = And(x=w558, y=w557) -> (x .and. y?=w546:bool)
          n223 = Insert Into Array(array=w548, new element=w551) -> (w549:dbl[])  [unwired: 1 in]
          n224 = Insert Into Array(array=w539, new element=w538) -> (w540:i32[])  [unwired: 1 in]
          n225 = Greater?(x=w542, y=w545) -> (0:w544:bool)
          n226 = Or(x=w546, y=w544) -> (x .or. y?=w543:bool)
          n227 = Insert Into Array(array=w535, new element=w534) -> (w536:i32[])  [unwired: 1 in]
          n228 = local write "tela"(w532) -> ()
          n229 = Index Array(array=w547, index=w542) -> (element=→"ponto_final":dbl)
          n230 = call-poly <vilib>:"Set Cursor.vi"() -> ()  [unwired: 10 in, 2 out]
        }
        "Array_x" <- w511
        "Horizontal_posicao_px" <- w508
        "Vertical_posicao_px" <- w507
        n231 = call-poly <vilib>:"Close Input Device.vi"("error in (no error)"=w521, "device ID"=w520) -> ()  [unwired: 8 in, 1 out]
        n232 = Subtract(x=w514, y=8 ("x")) -> (x-y=w512:i32)
        n233 = Multiply(x=w512, y=10) -> (x*y=→"Tempo de movimento":i32)
      }
      frame #10 {
        # "Isso serve para apagar"
        n234 = local read "Tempo de movimento"() -> (w587:i32)
        n235 = local read "Alvo_horizontal_px"() -> (w594:dbl)
        n236 = local read "Vertical_atual_px"() -> (w592:i32)
        n237 = local read "Horizontal_atual_px"() -> (w593:i32)
        n238 = local read "Alvo_vertical_px"() -> (w591:dbl)
        n239 = local read "Tempo de reação"() -> (w586:i32)
        n240 = while {
          tunnel: w617 -> [w656]
          shift-right: [w647] -> _
          shift-left: 0.0 -> [w648]
          shift-right: [w646] -> w611
          shift-left: dbl[] [] -> [w645]
          i -> [w651]
          stop <- w654 stop-if-true
          n241 = Increment(x=w651) -> (x+1=w658:i32)
          n242 = Array Size(array=w656) -> (size(s)=w657:i32)
          n243 = Index Array(array=w656, index=w658) -> (element=w650:i32)
          n244 = Index Array(array=w656, index=w651) -> (element=w653:i32)
          n245 = Subtract(x=w653, y=w650) -> (x-y=w649:i32)
          n246 = Decrement(x=w657) -> (x-1=w655:i32)
          n247 = Absolute Value(x=w649) -> (abs(x)=w652:i32)
          n248 = Equal?(x=w655, y=w651) -> (x = y?=w654:bool)
          n249 = Add(x=w648, y=w652) -> (x+y=w647:dbl)
          n250 = Insert Into Array(array=w645, new element=w647) -> (w646:dbl[])  [unwired: 1 in]
        }
        n251 = Add(x=w587, y=w586) -> (x+y=w585:i32)
        n252 = while {
          tunnel: w614 -> [w642]
          shift-right: [w633] -> _
          shift-left: 0.0 -> [w634]
          shift-right: [w632] -> w613
          shift-left: dbl[] [] -> [w631]
          i -> [w637]
          stop <- w640 stop-if-true
          n253 = Increment(x=w637) -> (x+1=w644:i32)
          n254 = Array Size(array=w642) -> (size(s)=w643:i32)
          n255 = Index Array(array=w642, index=w644) -> (element=w636:i32)
          n256 = Index Array(array=w642, index=w637) -> (element=w639:i32)
          n257 = Subtract(x=w639, y=w636) -> (x-y=w635:i32)
          n258 = Decrement(x=w643) -> (x-1=w641:i32)
          n259 = Absolute Value(x=w635) -> (abs(x)=w638:i32)
          n260 = Equal?(x=w641, y=w637) -> (x = y?=w640:bool)
          n261 = Add(x=w634, y=w638) -> (x+y=w633:dbl)
          n262 = Insert Into Array(array=w631, new element=w633) -> (w632:dbl[])  [unwired: 1 in]
        }
        n263 = Subtract(x=w591, y=w592) -> (x-y=w596:dbl)
        n264 = Number To Decimal String(number=w585) -> (decimal integer string=w603:string)  [unwired: 1 in]
        n265 = Subtract(x=w593, y=w594) -> (x-y=w595:dbl)
        n266 = local write "TM"(w603) -> ()
        n267 = Square(x=w596) -> (x^2=w598:dbl)
        n268 = property on="TM" class="Str"("Visible"=TRUE) -> ()  [unwired: 2 in, 2 out]
        n269 = Square(x=w595) -> (x^2=w597:dbl)
        n270 = case shown="True" TRUE {
          frame False {
          }
          frame True {
            n271 = Get Date/Time In Seconds() -> (seconds since 1Jan1904=w624:timestamp)
            n272 = Format Date/Time String(time format string (%c)="%H%M%S%4u", seconds (now)=w624) -> (date/time string=w628:string)  [unwired: 1 in]
            n273 = Fract/Exp String To Number(use system decimal point (T)=TRUE, string=w628) -> (number=w626:dbl)  [unwired: 2 in, 1 out]
            n274 = Subtract(x=w626, y=0.08) -> (x-y=→"Fim_resp":dbl)
            n275 = Seconds To Date/Time(time stamp (now)=w624) -> (date time rec=→"Fim_resp_Cluter":T1)  [unwired: 1 in]
          }
        }
        n276 = local read "Horizontal (cm/px)"() -> (w600:dbl)
        n277 = Add(x=w597, y=w598) -> (x+y=w599:dbl)
        n278 = local read "Horizontal (cm/px)"() -> (w610:dbl)
        n279 = Square Root(x=w599) -> (sqrt(x)=w601:dbl)
        n280 = local read "Horizontal (cm/px)"() -> (w612:dbl)
        n281 = property on="ER" class="Str"("Visible"=TRUE) -> ()  [unwired: 2 in, 2 out]
        n282 = Multiply(x=w601, y=w600) -> (x*y=w590:dbl)
        "erro radial (cm)" <- w590
        n283 = Multiply(x=w613, y=w612) -> (x*y=w609:dbl[])
        n284 = Multiply(x=w611, y=w610) -> (x*y=w608:dbl[])
        n285 = Format Value(format string="%.2f", value (0)=w590) -> (output string=w589:string)  [unwired: 1 in]
        n286 = call <vilib>:"Draw Circle by Radius.vi"() -> ("new picture"=w606:picture)  [unwired: 11 in]
        n287 = Square(x=w608) -> (x^2=w621:dbl[])
        n288 = Square(x=w609) -> (x^2=w620:dbl[])
        n289 = Add(x=w621, y=w620) -> (x+y=w622:dbl[])
        n290 = local write "ER"(w589) -> ()
        n291 = Square Root(x=w622) -> (sqrt(x)=w607:dbl[])
        n292 = local write "tela"(w606) -> ()
      }
      frame #11 {
        # "intervalor\nentre fim e o inicio"
        # "cortar o vetor"
        n293 = local read "Array_x"() -> (w673:dbl[])
        n294 = Array Size(array=w669) -> (size(s)=w671:i32)
        n295 = Array Size(array=w663) -> (size(s)=w667:i32)
        n296 = Array Size(array=w662) -> (size(s)=w683:i32)
        n297 = Array Size(array=w673) -> (size(s)=w678:i32)
        n298 = Subtract(x=w671, y=8) -> (x-y=w668:i32)
        n299 = Subtract(x=w667, y=8) -> (x-y=w665:i32)
        n300 = Wait (ms)(milliseconds to wait="Intervalo entre o fim e o inicio da próxima tentativa") -> ()  [unwired: 1 out]
        n301 = Subtract(x=w683, y=8) -> (x-y=w681:i32)
        n302 = Subtract(x=w678, y=8) -> (x-y=w676:i32)
        n303 = Array Subset(array=w669, index=2, length=w668) -> (w661:dbl[])
        "posicao_horizontal" <- w661
        n304 = Array Subset(array=w663, index=1, length=w665) -> (w660:dbl[])
        "posicao_vertical" <- w660
        n305 = Array Subset(array=w662, index=1, length=w681) -> (w680:dbl[])
        "posicao_total" <- w680
        n306 = Array Subset(array=w673, index=1, length=w676) -> (→"eixo x":dbl[])
      }
      frame #12 {
        n307 = Array Subset(array=w684, index=0, length=1) -> (w685:dbl[])
        n308 = Array Subset(array=w686, index=0, length=1) -> (w691:dbl[])
        n309 = Array Subset(array=w699, index=0, length=1) -> (w697:dbl[])
        n310 = Index Array(array=w685, index=0) -> (element=→"ref_p_inicial_horizontal":dbl)
        n311 = Index Array(array=w691, index=0) -> (element=→"ref_p_inicial_vertical":dbl)
        n312 = Index Array(array=w697, index=0) -> (element=→"ref_p_inicial_total":dbl)
      }
      frame #13 {
        # "Filtro"
        # "Filtro"
        n313 = local read "ref_p_inicial_total"() -> (w730:dbl)
        n314 = local read "ref_p_inicial_horizontal"() -> (w724:dbl)
        n315 = local read "ref_p_inicial_vertical"() -> (w727:dbl)
        n316 = Subtract(x=w725, y=w724) -> (x-y=w726:dbl[])
        n317 = Subtract(x=w731, y=w730) -> (x-y=w732:dbl[])
        n318 = Absolute Value(x=w726) -> (abs(x)=w714:dbl[])
        n319 = Subtract(x=w728, y=w727) -> (x-y=w729:dbl[])
        n320 = Absolute Value(x=w732) -> (abs(x)=w721:dbl[])
        n321 = Absolute Value(x=w729) -> (abs(x)=w717:dbl[])
        n322 = Array Size(array=w721) -> (size(s)=w723:i32)
        n323 = Array Size(array=w717) -> (size(s)=w719:i32)
        n324 = Array Size(array=w714) -> (size(s)=w716:i32)
        n325 = Array Subset(array=w721, index=1, length=w723) -> (→"Deslocamento_Total__bruto":dbl[])
        n326 = Array Subset(array=w717, index=1, length=w719) -> (w709:dbl[])
        "Deslocamento_Vertical_bruto" <- w709
        n327 = Array Subset(array=w714, index=1, length=w716) -> (w703:dbl[])
        "Deslocamento_Horizontal_bruto" <- w703
        n328 = call-poly <vilib>:"Butterworth Filter.vi"("order"=2, "filter type"=Filter_Passband_Type."Lowpass", "low cutoff freq: fl"=12.0, "sampling freq: fs"=100.0, "X"=w709) -> ("Filtered X"=→"Deslocamento_Vertical_fill":dbl[])  [unwired: 3 in, 1 out]
        n329 = call-poly <vilib>:"Butterworth Filter.vi"("order"=2, "filter type"=Filter_Passband_Type."Lowpass", "low cutoff freq: fl"=12.0, "sampling freq: fs"=100.0, "X"=w703) -> ("Filtered X"=→"Deslocamento_Horizontal_fill":dbl[])  [unwired: 3 in, 1 out]
      }
      frame #14 {
        # "fazendo a meta precisao"
        # "Filtro"
        n330 = local read "posicao_horizontal"() -> (w738:dbl[])
        n331 = local read "posicao_total"() -> (w737:dbl[])
        n332 = local read "Deslocamento_Total__bruto"() -> (w746:dbl[])
        n333 = local read "ref_V_alvo"() -> (w733:dbl)
        n334 = Divide(x=w738, y=w737) -> (x/y=w736:dbl[])
        n335 = local read "ref_H_alvo"() -> (w741:dbl)
        n336 = call <vilib>:"Draw Circle by Radius.vi"() -> ("new picture"=w740:picture)  [unwired: 11 in]
        n337 = Inverse Sine(1:w736) -> (0:w735:dbl[])
        n338 = call-poly <vilib>:"Butterworth Filter.vi"("order"=2, "filter type"=Filter_Passband_Type."Lowpass", "low cutoff freq: fl"=12.0, "sampling freq: fs"=100.0, "X"=w746) -> ("Filtered X"=→"Deslocamento_total_filtrado":dbl[])  [unwired: 3 in, 1 out]
        n339 = Square(x=w733) -> (x^2=w743:dbl)
        n340 = Square(x=w741) -> (x^2=w742:dbl)
        n341 = local write "tela"(w740) -> ()
        n342 = expression code="(x/pi)*180.0" "radians to degrees"(w735) -> (→"Graus":dbl[])
        n343 = Add(x=w742, y=w743) -> (x+y=w744:dbl)
        n344 = Square Root(x=w744) -> (sqrt(x)=→"meta_precisao":dbl)
      }
      frame #15 {
        n345 = local read "Deslocamento_total_filtrado"() -> (w751:dbl[])
        n346 = local read "eixo x"() -> (w752:dbl[])
        n347 = call "Convert to Dynamic Data"("Array"=w752) -> ("Dynamic Data Type"=w753:dynamicdata)  [unwired: 3 in]
        n348 = call "Convert to Dynamic Data2"("Array"=w751) -> ("Dynamic Data Type"=w754:dynamicdata)  [unwired: 3 in]
        n349 = call "deslocamento"("Y Input"=w754, "X Input"=w753) -> ("XY Graph"=→"Deslocamento":cluster{"X":dbl[], "Y":dbl[]}[])  [unwired: 8 in, 1 out]
      }
      frame #16 {
        # "Velocidade"
        # "Velocidade"
        n350 = local read "Deslocamento_total_filtrado"() -> (w772:dbl[])
        n351 = call <vilib>:"Derivative x(t).vi"("dt"=0.01, "Initial Condition"=dbl[] [0.0], "X"=w772) -> ("dX/dt"=w756:dbl[])  [unwired: 7 in, 1 out]
        n352 = local read "eixo x"() -> (w757:dbl[])
        n353 = call-poly <vilib>:"Butterworth Filter.vi"("order"=2, "filter type"=Filter_Passband_Type."Lowpass", "low cutoff freq: fl"=12.0, "sampling freq: fs"=100.0, "X"=w756) -> ("Filtered X"=w758:dbl[])  [unwired: 3 in, 1 out]
        n354 = Array Size(array=w758) -> (size(s)=w766:i32)
        n355 = call "Convert to Dynamic Data3"("Array"=w757) -> ("Dynamic Data Type"=w770:dynamicdata)  [unwired: 3 in]
        n356 = Subtract(x=w766, y=1) -> (x-y=w764:i32)
        n357 = Array Subset(array=w758, index=0, length=w764) -> (w763:dbl[])
        "Velocidade" <- w763
        n358 = call "Convert to Dynamic Data4"("Array"=w763) -> ("Dynamic Data Type"=w769:dynamicdata)  [unwired: 3 in]
        n359 = call "velocidade"("Y Input"=w769, "X Input"=w770) -> ("XY Graph"=→"Velocidade":cluster{"X":dbl[], "Y":dbl[]}[])  [unwired: 8 in, 1 out]
      }
      frame #17 {
        # "Filtro"
        # "Aceleracao"
        # "Acelracao"
        n360 = local read "Velocidade"() -> (w786:dbl[])
        n361 = call <vilib>:"Derivative x(t).vi"("dt"=0.01, "Initial Condition"=dbl[] [0.0], "X"=w786) -> ("dX/dt"=w775:dbl[])  [unwired: 7 in, 1 out]
        n362 = call-poly <vilib>:"Butterworth Filter.vi"("order"=2, "filter type"=Filter_Passband_Type."Lowpass", "low cutoff freq: fl"=12.0, "sampling freq: fs"=100.0, "X"=w775) -> ("Filtered X"=w774:dbl[])  [unwired: 3 in, 1 out]
        n363 = local read "eixo x"() -> (w787:dbl[])
        n364 = call "Convert to Dynamic Data6"("Array"=w787) -> ("Dynamic Data Type"=w791:dynamicdata)  [unwired: 3 in]
        n365 = Array Size(array=w774) -> (size(s)=w783:i32)
        n366 = Subtract(x=w783, y=2) -> (x-y=w781:i32)
        n367 = Array Subset(array=w774, index=0, length=w781) -> (w780:dbl[])
        "aceleracao" <- w780
        n368 = call "Convert to Dynamic Data5"("Array"=w780) -> ("Dynamic Data Type"=w790:dynamicdata)  [unwired: 3 in]
        n369 = call "aceleracao"("Y Input"=w790, "X Input"=w791) -> ("XY Graph"=→"Aceleracao":cluster{"X":dbl[], "Y":dbl[]}[])  [unwired: 8 in, 1 out]
      }
      frame #18 {
        # "jeark"
        n370 = local read "aceleracao"() -> (w805:dbl[])
        n371 = call <vilib>:"Derivative x(t).vi"("dt"=0.01, "Initial Condition"=dbl[] [0.0], "X"=w805) -> ("dX/dt"=w793:dbl[])  [unwired: 7 in, 1 out]
        n372 = local read "eixo x"() -> (w804:dbl[])
        n373 = call-poly <vilib>:"Butterworth Filter.vi"("order"=2, "filter type"=Filter_Passband_Type."Lowpass", "low cutoff freq: fl"=12.0, "sampling freq: fs"=100.0, "X"=w793) -> ("Filtered X"=w792:dbl[])  [unwired: 3 in, 1 out]
        n374 = Array Size(array=w792) -> (size(s)=w802:i32)
        n375 = Subtract(x=w802, y=3) -> (x-y=w800:i32)
        n376 = Array Subset(array=w792, index=0, length=w800) -> (w799:dbl[])
        "Jeark" <- w799
        n377 = call "Convert to Dynamic Data8"("Array"=w804) -> ("Dynamic Data Type"=w808:dynamicdata)  [unwired: 3 in]
        n378 = call "Convert to Dynamic Data7"("Array"=w799) -> ("Dynamic Data Type"=w794:dynamicdata)  [unwired: 3 in]
        n379 = call "jeark"("Y Input"=w794, "X Input"=w808) -> ("XY Graph"=→"Jeark":cluster{"X":dbl[], "Y":dbl[]}[])  [unwired: 8 in, 1 out]
      }
      frame #19 {
        n380 = local read "Velocidade"() -> (w812:dbl[])
        n381 = call "Convert to Dynamic Data25"("Array"=w812) -> ("Dynamic Data Type"=w811:dynamicdata)  [unwired: 3 in]
        n382 = call "Statistics"("Signals"=w811) -> ("Maximum"=→"Pico_velocidade":dynamicdata)  [unwired: 25 in, 1 out]
      }
      frame #20 {
        n383 = local read "aceleracao"() -> (w813:dbl[])
        n384 = while {
          tunnel: w813 -> [w821]
          shift-right: [w818] -> w814
          shift-left: i32[] [] -> [w817]
          i -> [w820]
          stop <- w816 stop-if-true
          w826 = 0.0 ("y")
          w830 = 0.0 ("y")
          n385 = Add(x=1, y=w820) -> (x+y=w834:i32)
          n386 = Index Array(array=w821, index=w834) -> (element=w827:dbl)
          n387 = Index Array(array=w821, index=w820) -> (element=w828:dbl)
          n388 = Less Or Equal?(x=w827, y=w830) -> (x <= y?=w832:bool)
          n389 = Greater Or Equal?(x=w827, y=w826) -> (x >= y?=w824:bool)
          n390 = Greater?(x=w828, y=w830) -> (0:w829:bool)
          n391 = Less?(x=w828, y=w826) -> (x < y?=w825:bool)
          n392 = And(x=w829, y=w832) -> (x .and. y?=w831:bool)
          n393 = And(x=w825, y=w824) -> (x .and. y?=w823:bool)
          n394 = Or(x=w831, y=w823) -> (x .or. y?=w822:bool)
          n395 = Array Size(array=w821) -> (size(s)=w819:i32)
          n396 = case shown="True" w822 {
            tunnel: w820 -> [_ w838]
            tunnel: [w835 w837] -> w818
            tunnel: w817 -> [w835 w836]
            frame False {
            }
            frame True {
              n397 = while {
                tunnel: w838 -> [w839]
                tunnel: [w842] -> w837
                tunnel: w836 -> [w843]
                i -> [w846]
                stop <- w844 stop-if-true
                n398 = Add(x=w839, y=2) -> (x+y=w840:i32)
                n399 = Equal?(x=1, y=w846) -> (x = y?=w844:bool)
                n400 = Insert Into Array(array=w843, new element=w840) -> (w842:i32[])  [unwired: 1 in]
              }
            }
          }
          n401 = Greater?(x=w820, y=w819) -> (0:w816:bool)
        }
        "ref_zero_cross" <- w814
      }
      frame #21 {
        # "posicao final em graus"
        # "Segundo ponto de correção"
        n402 = local read "Deslocamento_Vertical_fill"() -> (w848:dbl[])
        n403 = local read "ref_zero_cross"() -> (w885:i32[])
        n404 = local read "Deslocamento_total_filtrado"() -> (w863:dbl[])
        n405 = local read "Deslocamento_Horizontal_fill"() -> (w847:dbl[])
        n406 = local read "Graus"() -> (w872:dbl[])
        n407 = Array Size(array=w848) -> (size(s)=w862:i32)
        n408 = Array Size(array=w885) -> (size(s)=w884:i32)
        n409 = Array Size(array=w863) -> (size(s)=w871:i32)
        n410 = Subtract(x=w862, y=1) -> (x-y=w860:i32)
        n411 = Subtract(x=w884, y=1) -> (x-y=w882:i32)
        n412 = Array Size(array=w847) -> (size(s)=w855:i32)
        n413 = Subtract(x=w871, y=1) -> (x-y=w869:i32)
        n414 = Array Size(array=w872) -> (size(s)=w878:i32)
        n415 = Array Subset(array=w885, index=1, length=1) -> (w888:i32[])
        n416 = Array Subset(array=w848, index=w860, length=1) -> (w857:dbl[])
        n417 = Array Subset(array=w885, index=2, length=w882) -> (w881:i32[])
        n418 = Subtract(x=w855, y=1) -> (x-y=w853:i32)
        n419 = Array Subset(array=w863, index=w869, length=1) -> (w866:dbl[])
        n420 = Subtract(x=w878, y=1) -> (x-y=w876:i32)
        n421 = Index Array(array=w888, index=0) -> (element=w864:i32)
        n422 = Index Array(array=w857, index=0) -> (element=→"Posicao_final_Vertical":dbl)
        n423 = Array Subset(array=w847, index=w853, length=1) -> (w850:dbl[])
        n424 = Array Subset(array=w872, index=w876, length=1) -> (w874:dbl[])
        n425 = Multiply(x=w864, y=10) -> (x*y=→"Tempo_para_o_pico":i32)
        n426 = Index Array(array=w866, index=0) -> (element=→"Posicao_cm_final":dbl)
        n427 = Array Size(array=w881) -> (size(s)=→"n_correcoes":i32)
        n428 = Index Array(array=w874, index=0) -> (element=→"Posicao_graus_final":dbl)
        n429 = Index Array(array=w850, index=0) -> (element=→"Posicao_final_horizontal":dbl)
      }
      frame #22 {
        n430 = local read "Deslocamento_total_filtrado"() -> (w902:dbl[])
        n431 = local read "Deslocamento_Vertical_fill"() -> (w918:dbl[])
        n432 = local read "Tempo_para_o_pico"() -> (w927:i32)
        n433 = local read "Horizontal (cm/px)"() -> (w930:dbl)
        n434 = local read "Deslocamento_Horizontal_fill"() -> (w913:dbl[])
        n435 = local read "Tempo_para_o_pico"() -> (w931:i32)
        n436 = local read "meta_precisao"() -> (w929:dbl)
        n437 = local read "Graus"() -> (w933:dbl[])
        n438 = local read "Tempo de movimento"() -> (w948:i32)
        n439 = Array Subset(array=w902, index=w900, length=1) -> (w922:dbl[])
        n440 = local read "aceleracao"() -> (w907:dbl[])
        n441 = local read "Inicio_da_resposta"() -> (w925:dbl)
        n442 = local read "aceleracao"() -> (w899:dbl[])
        n443 = Index Array(array=w922, index=0) -> (element=w941:dbl)
        n444 = Array Size(array=w902) -> (size(s)=w903:i32)
        n445 = Array Subset(array=w933, index=w912, length=1) -> (w935:dbl[])
        n446 = Array Size(array=w907) -> (size(s)=w906:i32)
        n447 = Array Subset(array=w902, index=w912, length=1) -> (w939:dbl[])
        n448 = Multiply(x=w929, y=w930) -> (x*y=w928:dbl)
        n449 = Multiply(x=w931, y=100) -> (x*y=w947:i32)
        n450 = Divide(x=w927, y=1000) -> (x/y=w924:dbl)
        n451 = Subtract(x=w941, y=w928) -> (x-y=w943:dbl)
        n452 = Index Array(array=w935, index=0) -> (element=→"Posicao_graus_2_sub":dbl)
        n453 = Array Subset(array=w907, index=w900, length=w906) -> (w905:dbl[])
        n454 = Index Array(array=w939, index=0) -> (element=→"Posicao_cm_2_sub":dbl)
        n455 = Absolute Value(x=w943) -> (abs(x)=→"ER_no_2_sub":dbl)
        n456 = Divide(x=w947, y=w948) -> (x/y=→"Tempo_relativo_pico":dbl)
        n457 = Array Subset(array=w913, index=w912, length=1) -> (w910:dbl[])
        n458 = Array Subset(array=w899, index=0, length=w900) -> (w897:dbl[])
        n459 = Array Subset(array=w902, index=w900, length=w903) -> (→"Deslocamento_tototal_2_sub":dbl[])
        n460 = Array Subset(array=w918, index=w912, length=1) -> (w915:dbl[])
        n461 = Add(x=w925, y=w924) -> (x+y=→"2_sub_mov":dbl)
        n462 = Array Subset(array=w902, index=0, length=w900) -> (→"Deslocamento_tototal_1_sub":dbl[])
        n463 = call-poly <vilib>:"Numeric Integration.vi"("dt"=0.01, "Input Array"=w905) -> ("result"=w894:dbl)  [unwired: 1 in, 1 out]
        n464 = Index Array(array=w910, index=0) -> (element=→"Posicao_Hori_2_sub":dbl)
        n465 = Absolute Value(x=w894) -> (abs(x)=→"Area_acel_2_sub":dbl)
        n466 = Index Array(array=w915, index=0) -> (element=→"Posicao_vert_2_sub":dbl)
        n467 = call-poly <vilib>:"Numeric Integration.vi"("dt"=0.01, "Input Array"=w897) -> ("result"=w896:dbl)  [unwired: 1 in, 1 out]
        n468 = Absolute Value(x=w896) -> (abs(x)=→"Area_acel_1_sub":dbl)
      }
      frame #23 {
        w1058 = ".txt" ("string")
        n469 = local read "Deslocamento_tototal_2_sub"() -> (w963:dbl[])
        n470 = local read "Fim_do_warning_Cluter"() -> (w1000:T1)
        n471 = local read "Inicio_da_resposta_Cluter"() -> (w982:T1)
        n472 = local read "Deslocamento_tototal_1_sub"() -> (w965:dbl[])
        n473 = local read "posicao_total"() -> (w1034:dbl[])
        n474 = local read "Deslocamento_Horizontal_bruto"() -> (w1031:dbl[])
        n475 = local read "posicao_vertical"() -> (w1033:dbl[])
        n476 = local read "Velocidade"() -> (w1036:dbl[])
        n477 = local read "Deslocamento_Vertical_bruto"() -> (w1032:dbl[])
        n478 = local read "Inicio_do_warning_Cluter"() -> (w1009:T1)
        n479 = local read "Deslocamento_total_filtrado"() -> (w1054:dbl[])
        n480 = local read "aceleracao"() -> (w1035:dbl[])
        n481 = local read "Deslocamento_Total__bruto"() -> (w1044:dbl[])
        n482 = local read "Digite aqui o endereço e nome do arquivo"() -> (w953:string)
        n483 = local read "posicao_horizontal"() -> (w1046:dbl[])
        n484 = local read "Jeark"() -> (w1050:dbl[])
        n485 = local read "Tempo_para_o_pico"() -> (w968:i32)
        n486 = local read "tentativa"() -> (w1055:i32)
        n487 = local read "Vertical_posicao_px"() -> (w1040:i32[])
        n488 = local read "Horizontal_posicao_px"() -> (w1038:i32[])
        n489 = local read "Graus"() -> (w1028:dbl[])
        n490 = local read "Apresentacao_do_estimulo_Cluter"() -> (w991:T1)
        n491 = Unbundle(w982) -> ("fractional second"=w988:dbl, "second"=w987:i32, "minute"=w990:i32, "hour"=w984:i32)  [unwired: 6 out]
        n492 = Concatenate Strings(w953, "_tentativa_" ("string")) -> (w1029:string)
        n493 = Unbundle(w1000) -> ("fractional second"=w1006:dbl, "second"=w1005:i32, "minute"=w1008:i32, "hour"=w1002:i32)  [unwired: 6 out]
        n494 = Format Into String(w1055) -> (resulting string=w1059:string)  [unwired: 3 in, 1 out]
        n495 = Multiply(x=w990, y=60) -> (x*y=w986:i32)
        n496 = Divide(x=w968, y=1000) -> (x/y=w966:dbl)
        n497 = Multiply(x=w984, y=3600) -> (x*y=w985:i32)
        n498 = Unbundle(w1009) -> ("fractional second"=w1015:dbl, "second"=w1014:i32, "minute"=w1017:i32, "hour"=w1011:i32)  [unwired: 6 out]
        n499 = local read "INICIO_Cluter"() -> (w1020:T1)
        n500 = Concatenate Strings(w1029, w1059) -> (w950:string)
        n501 = Multiply(x=w1008, y=60) -> (x*y=w1004:i32)
        n502 = Multiply(x=w1002, y=3600) -> (x*y=w1003:i32)
        n503 = Compound Arithmetic op=ADD(w988, w987, w986, w985) -> (w967:dbl)
        "Inicio_da_reposta(s)" <- w967
        n504 = call "Convert to Dynamic Data9"("Array"=w1054) -> ("Dynamic Data Type"=w1053:dynamicdata)  [unwired: 3 in]
        n505 = call "Convert to Dynamic Data15"("Array"=w1035) -> ("Dynamic Data Type"=w1051:dynamicdata)  [unwired: 3 in]
        n506 = call "Convert to Dynamic Data16"("Array"=w1050) -> ("Dynamic Data Type"=w1049:dynamicdata)  [unwired: 3 in]
        n507 = call "Convert to Dynamic Data14"("Array"=w1036) -> ("Dynamic Data Type"=w1052:dynamicdata)  [unwired: 3 in]
        n508 = call "Convert to Dynamic Data18"("Array"=w1033) -> ("Dynamic Data Type"=w1047:dynamicdata)  [unwired: 3 in]
        n509 = call "Convert to Dynamic Data19"("Array"=w1046) -> ("Dynamic Data Type"=w1045:dynamicdata)  [unwired: 3 in]
        n510 = Multiply(x=w1017, y=60) -> (x*y=w1013:i32)
        n511 = local read "Fim_resp_Cluter"() -> (w974:T1)
        n512 = call "Convert to Dynamic Data17"("Array"=w1034) -> ("Dynamic Data Type"=w1048:dynamicdata)  [unwired: 3 in]
        n513 = call "Convert to Dynamic Data20"("Array"=w1044) -> ("Dynamic Data Type"=w1043:dynamicdata)  [unwired: 3 in]
        n514 = Multiply(x=w1011, y=3600) -> (x*y=w1012:i32)
        n515 = Concatenate Strings(w950, w1058) -> (w1057:string)
        n516 = Compound Arithmetic op=ADD(w1006, w1005, w1004, w1003) -> (→"Fim_do_warning(s)":dbl)
        n517 = call "Convert to Dynamic Data21"("Array"=w1032) -> ("Dynamic Data Type"=w1042:dynamicdata)  [unwired: 3 in]
        n518 = Add(x=w967, y=w966) -> (x+y=→"2_sub_mov(s)":dbl)
        n519 = Concatenate Strings(w953, w1058) -> (w1056:string)
        n520 = call "Convert to Dynamic Data22"("Array"=w1031) -> ("Dynamic Data Type"=w1041:dynamicdata)  [unwired: 3 in]
        n521 = call "Convert to Dynamic Data23"("Array"=w1040) -> ("Dynamic Data Type"=w1039:dynamicdata)  [unwired: 3 in]
        n522 = call "Convert to Dynamic Data24"("Array"=w1038) -> ("Dynamic Data Type"=w1037:dynamicdata)  [unwired: 3 in]
        n523 = Compound Arithmetic op=ADD(w1015, w1014, w1013, w1012) -> (→"Inicio_do_warning(s)":dbl)
        n524 = String To Path(string=w1056) -> (path=→"referencia de endereco":path)
        n525 = call "Convert to Dynamic Data29"("Array"=w1028) -> ("Dynamic Data Type"=w1027:dynamicdata)  [unwired: 3 in]
        n526 = Unbundle(w1020) -> ("fractional second"=w1024:dbl, "second"=w1023:i32, "minute"=w1026:i32, "hour"=w1019:i32)  [unwired: 6 out]
        n527 = String To Path(string=w1057) -> (path=w1060:path)
        n528 = Unbundle(w991) -> ("fractional second"=w997:dbl, "second"=w996:i32, "minute"=w999:i32, "hour"=w993:i32)  [unwired: 6 out]
        n529 = Unbundle(w974) -> ("fractional second"=w979:dbl, "second"=w961:i32, "minute"=w981:i32, "hour"=w976:i32)  [unwired: 6 out]
        n530 = call "Convert to Dynamic Data51"("Array"=w963) -> ("Dynamic Data Type"=w962:dynamicdata)  [unwired: 3 in]
        n531 = call "Convert to Dynamic Data50"("Array"=w965) -> ("Dynamic Data Type"=w964:dynamicdata)  [unwired: 3 in]
        n532 = Concatenate Strings(w950, ".xls" ("string")) -> (w956:string)
        n533 = Multiply(x=w1026, y=60) -> (x*y=w1022:i32)
        n534 = Multiply(x=w999, y=60) -> (x*y=w995:i32)
        n535 = Multiply(x=w1019, y=3600) -> (x*y=w1021:i32)
        n536 = Multiply(x=w993, y=3600) -> (x*y=w994:i32)
        n537 = Merge Signals(w1053, w1052, w1051, w1049, w1048, w1047, w1045, w1043, w1042, w1041, w1039, w1037, w1027, w964, w962) -> (w954:dynamicdata)
        n538 = Multiply(x=w981, y=60) -> (x*y=w978:i32)
        n539 = Multiply(x=w976, y=3600) -> (x*y=w977:i32)
        n540 = String To Path(string=w956) -> (path=w955:path)
        n541 = Compound Arithmetic op=ADD(w1024, w1023, w1022, w1021) -> (→"INICIO(s)":dbl)
        n542 = Compound Arithmetic op=ADD(w997, w996, w995, w994) -> (→"Apresentacao_do_estimulo(s)":dbl)
        n543 = Compound Arithmetic op=ADD(w979, w961, w978, w977) -> (w958:dbl)
        n544 = call "Salvar em xls"("Signals"=w954, "Filename"=w955) -> ()  [unwired: 15 in, 3 out]
        n545 = call "Salvar em txt"("Signals"=w954, "Filename"=w1060) -> ()  [unwired: 15 in, 3 out]
        n546 = Subtract(x=w958, y=0.08) -> (x-y=→"Fim_da_reposta(s)":dbl)
      }
      frame #24 {
        n547 = local read "Horizontal (cm/px)"() -> (w1074:dbl)
        n548 = local read "Horizontal"() -> (w1070:dbl)
        n549 = local read "ref_V_alvo"() -> (w1075:dbl)
        n550 = local read "ref_H_alvo"() -> (w1076:dbl)
        n551 = local read "Apresentacao_do_estimulo"() -> (w1093:dbl)
        n552 = local read "Apresentacao_do_estimulo(s)"() -> (w1086:dbl)
        n553 = local read "Inicio_da_reposta(s)"() -> (w1085:dbl)
        n554 = local read "Area_acel_2_sub"() -> (w1078:dbl)
        n555 = local read "Posicao_final_horizontal"() -> (w1082:dbl)
        n556 = local read "Inicio_do_warning(s)"() -> (w1088:dbl)
        n557 = local read "Inicio_da_resposta"() -> (w1092:dbl)
        n558 = local read "Fim_do_warning(s)"() -> (w1087:dbl)
        n559 = local read "Vertical  (cm)"() -> (w1073:dbl)
        n560 = local read "Fim_do_warning"() -> (w1094:dbl)
        n561 = local read "Posicao_final_Vertical"() -> (w1081:dbl)
        n562 = local read "Horizontal_atual_px"() -> (w1064:i32)
        n563 = local read "Fim_da_reposta(s)"() -> (w1083:dbl)
        n564 = local read "Alvo_horizontal_px"() -> (w1062:dbl)
        n565 = local read "Inicio_do_warning"() -> (w1095:dbl)
        n566 = local read "Tempo de movimento"() -> (w1108:i32)
        n567 = local read "Vertical_atual_px"() -> (w1063:i32)
        n568 = local read "Tempo de reação"() -> (w1109:i32)
        n569 = local read "INICIO"() -> (w1096:dbl)
        n570 = local read "2_sub_mov(s)"() -> (w1084:dbl)
        n571 = local read "Posicao_Hori_2_sub"() -> (w1080:dbl)
        n572 = local read "2_sub_mov"() -> (w1091:dbl)
        n573 = local read "Alvo_vertical_px"() -> (w1061:dbl)
        n574 = local read "INICIO(s)"() -> (w1089:dbl)
        n575 = local read "Tempo_relativo_pico"() -> (w1105:dbl)
        n576 = local read "Posicao_graus_2_sub"() -> (w1098:dbl)
        n577 = local read "Posicao_cm_final"() -> (w1101:dbl)
        n578 = local read "Tempo_para_o_pico"() -> (w1097:i32)
        n579 = local read "Posicao_vert_2_sub"() -> (w1079:dbl)
        n580 = local read "Posicao_cm_2_sub"() -> (w1099:dbl)
        n581 = local read "Pico_velocidade"() -> (w1104:dbl)
        n582 = local read "Posicao_graus_final"() -> (w1102:dbl)
        n583 = local read "erro radial (cm)"() -> (w1106:dbl)
        n584 = local read "ER_no_2_sub"() -> (w1100:dbl)
        n585 = local read "Area_acel_1_sub"() -> (w1077:dbl)
        n586 = local read "n_correcoes"() -> (w1103:i32)
        n587 = local read "Fim_resp"() -> (w1090:dbl)
        n588 = Multiply(x=w1076, y=w1074) -> (x*y=w1071:dbl)
        n589 = local read "Vertical"() -> (w1068:dbl)
        n590 = local read "codigo"() -> (w1065:dbl)
        n591 = Multiply(x=w1075, y=w1074) -> (x*y=w1072:dbl)
        n592 = Subtract(x=w1071, y=w1070) -> (x-y=w1069:dbl)
        n593 = Add(x=w1109, y=w1108) -> (x+y=w1107:i32)
        n594 = Subtract(x=w1073, y=w1072) -> (x-y=w1067:dbl)
        n595 = Subtract(x=w1067, y=w1068) -> (x-y=w1066:dbl)
      }
    }
  }
  n596 = call "Convert to Dynamic Data27"("Array"=w71) -> ("Dynamic Data Type"=w70:dynamicdata)  [unwired: 3 in]
  n597 = call "Convert to Dynamic Data13"("Array"=w75) -> ("Dynamic Data Type"=w74:dynamicdata)  [unwired: 3 in]
  n598 = call "Convert to Dynamic Data10"("Array"=w81) -> ("Dynamic Data Type"=w80:dynamicdata)  [unwired: 3 in]
  n599 = call "Convert to Dynamic Data12"("Array"=w77) -> ("Dynamic Data Type"=w76:dynamicdata)  [unwired: 3 in]
  n600 = call "Convert to Dynamic Data26"("Array"=w73) -> ("Dynamic Data Type"=w72:dynamicdata)  [unwired: 3 in]
  n601 = call "Convert to Dynamic Data30"("Array"=w67) -> ("Dynamic Data Type"=w66:dynamicdata)  [unwired: 3 in]
  n602 = call "Convert to Dynamic Data28"("Array"=w69) -> ("Dynamic Data Type"=w68:dynamicdata)  [unwired: 3 in]
  n603 = call "Convert to Dynamic Data11"("Array"=w79) -> ("Dynamic Data Type"=w78:dynamicdata)  [unwired: 3 in]
  n604 = call "Convert to Dynamic Data31"("Array"=w65) -> ("Dynamic Data Type"=w64:dynamicdata)  [unwired: 3 in]
  n605 = call "Convert to Dynamic Data33"("Array"=w61) -> ("Dynamic Data Type"=w60:dynamicdata)  [unwired: 3 in]
  n606 = call "Convert to Dynamic Data32"("Array"=w63) -> ("Dynamic Data Type"=w62:dynamicdata)  [unwired: 3 in]
  n607 = call "Convert to Dynamic Data34"("Array"=w59) -> ("Dynamic Data Type"=w58:dynamicdata)  [unwired: 3 in]
  n608 = call "Convert to Dynamic Data35"("Array"=w57) -> ("Dynamic Data Type"=w56:dynamicdata)  [unwired: 3 in]
  n609 = call "Convert to Dynamic Data37"("Array"=w52) -> ("Dynamic Data Type"=w53:dynamicdata)  [unwired: 3 in]
  n610 = call "Convert to Dynamic Data36"("Array"=w55) -> ("Dynamic Data Type"=w54:dynamicdata)  [unwired: 3 in]
  n611 = call "Convert to Dynamic Data38"("Array"=w51) -> ("Dynamic Data Type"=w50:dynamicdata)  [unwired: 3 in]
  n612 = call "Convert to Dynamic Data39"("Array"=w48) -> ("Dynamic Data Type"=w49:dynamicdata)  [unwired: 3 in]
  n613 = call "Convert to Dynamic Data40"("Array"=w47) -> ("Dynamic Data Type"=w46:dynamicdata)  [unwired: 3 in]
  n614 = call "Convert to Dynamic Data41"("Array"=w45) -> ("Dynamic Data Type"=w44:dynamicdata)  [unwired: 3 in]
  n615 = call "Convert to Dynamic Data42"("Array"=w43) -> ("Dynamic Data Type"=w42:dynamicdata)  [unwired: 3 in]
  n616 = call "Convert to Dynamic Data43"("Array"=w41) -> ("Dynamic Data Type"=w40:dynamicdata)  [unwired: 3 in]
  n617 = call "Convert to Dynamic Data44"("Array"=w39) -> ("Dynamic Data Type"=w38:dynamicdata)  [unwired: 3 in]
  n618 = call "Convert to Dynamic Data45"("Array"=w37) -> ("Dynamic Data Type"=w36:dynamicdata)  [unwired: 3 in]
  n619 = call "Convert to Dynamic Data47"("Array"=w32) -> ("Dynamic Data Type"=w33:dynamicdata)  [unwired: 3 in]
  n620 = call "Convert to Dynamic Data46"("Array"=w35) -> ("Dynamic Data Type"=w34:dynamicdata)  [unwired: 3 in]
  n621 = call "Convert to Dynamic Data48"("Array"=w30) -> ("Dynamic Data Type"=w31:dynamicdata)  [unwired: 3 in]
  n622 = call "Convert to Dynamic Data49"("Array"=w29) -> ("Dynamic Data Type"=w28:dynamicdata)  [unwired: 3 in]
  n623 = call "Convert to Dynamic Data52"("Array"=w27) -> ("Dynamic Data Type"=w21:dynamicdata)  [unwired: 3 in]
  n624 = call "Convert to Dynamic Data53"("Array"=w26) -> ("Dynamic Data Type"=w25:dynamicdata)  [unwired: 3 in]
  n625 = call "Convert to Dynamic Data54"("Array"=w24) -> ("Dynamic Data Type"=w23:dynamicdata)  [unwired: 3 in]
  n626 = call "Convert to Dynamic Data55"("Array"=w22) -> ("Dynamic Data Type"=w20:dynamicdata)  [unwired: 3 in]
  n627 = call "Convert to Dynamic Data56"("Array"=w13) -> ("Dynamic Data Type"=w14:dynamicdata)  [unwired: 3 in]
  n628 = call "Convert to Dynamic Data57"("Array"=w19) -> ("Dynamic Data Type"=w18:dynamicdata)  [unwired: 3 in]
  n629 = call "Convert to Dynamic Data58"("Array"=w17) -> ("Dynamic Data Type"=w12:dynamicdata)  [unwired: 3 in]
  n630 = call "Convert to Dynamic Data59"("Array"=w16) -> ("Dynamic Data Type"=w15:dynamicdata)  [unwired: 3 in]
  n631 = call "Convert to Dynamic Data60"("Array"=w9) -> ("Dynamic Data Type"=w11:dynamicdata)  [unwired: 3 in]
  n632 = call "Convert to Dynamic Data61"("Array"=w8) -> ("Dynamic Data Type"=w7:dynamicdata)  [unwired: 3 in]
  n633 = call "Convert to Dynamic Data62"("Array"=w6) -> ("Dynamic Data Type"=w5:dynamicdata)  [unwired: 3 in]
  n634 = call "Convert to Dynamic Data63"("Array"=w4) -> ("Dynamic Data Type"=w3:dynamicdata)  [unwired: 3 in]
  n635 = call "Convert to Dynamic Data64"("Array"=w2) -> ("Dynamic Data Type"=w1:dynamicdata)  [unwired: 3 in]
  n636 = Merge Signals(w80, w78, w76, w74, w72, w70, w68, w66, w64, w62, w60, w58, w56, w54, w53, w50, w49, w46, w44, w42, w40, w38, w36, w34, w33, w31, w28, w21, w25, w23, w20, w14, w18, w12, w15, w11, w7, w5, w3, w1) -> (w82:dynamicdata)
  n637 = call "Dados Brutos"("Signals"=w82) -> ("Table"=w84:string[][])  [unwired: 4 in, 6 out]
  n638 = Fract/Exp String To Number(string=w84) -> (number=w85:dbl[][])  [unwired: 3 in, 1 out]
  n639 = call-poly <vilib>:"Write Delimited Spreadsheet.vi"("format (%.3f)"="%.3f", "2D data"=w85) -> ()  [unwired: 12 in, 2 out]
